vi "Measurement Logic.vi"() -> ()   [LabVIEW 2021, in "PWM Dimming.lvlib"]
uses:
  PWM Dimming.lvlib
  <vilib>/Plug-In SDKs/Measurements/Measure Call Context/Measure Call Context.lvclass
  Measurement Configuration.ctl
  Measurement Results.ctl
  Sub-VI/PWM measurement data.ctl
  <instrlib>/niDCPower/nidcpower.llb/niDCPower Source Mode.ctl
  <instrlib>/niDCPower/nidcpower.llb/niDCPower Output Function.ctl
  <instrlib>/niDCPower/nidcpower.llb/niDCPower Wait For Event - Event.ctl
  <instrlib>/niFgen/niFgen.llb/niFgen Output Mode.ctl
  <instrlib>/niFgen/niFgen.llb/niFgen Waveform Type.ctl
  <instrlib>/niDCPower/nidcpower.llb/niDCPower Aperture Time Units.ctl
  <instrlib>/niDCPower/nidcpower.llb/niDCPower Export Signal - Signal.ctl
  <instrlib>/niScope/Controls/niScope trigger slope.ctl
  <instrlib>/niFgen/niFgen.llb/niFgen Disable Start Trigger.vi
  <instrlib>/niDCPower/nidcpower.llb/niDCPower Configure Digital Edge Source Trigger With Channels.vi
  <instrlib>/niDCPower/nidcpower.llb/niDCPower Configure Digital Edge Measure Trigger With Channels.vi
  <instrlib>/niFgen/niFgen.llb/niFgen Configure Digital Edge Start Trigger.vi
  <instrlib>/niScope/Utility/niScope Get Channel Name From String.vi
  <instrlib>/niScope/Configure/Trigger/niScope Configure Trigger Digital.vi
  <instrlib>/niScope/Acquire/Fetch/niScope Fetch WDT.vi
panel:
  out "measurement results":T1
  in  "measurement configuration":T2={"DUT setup time"=1.0, "Nominal output voltage"=3.3, "Duty cycle single pulse/sweep pulse"=TRUE, "PWM frequency"=25.0, "Start duty cycle"=0.9, "Stop duty cycle"=99.1, "Number of sweep points"=10, "Duty cycle sweep type"="Linear", "Duty cycle single point"=50.0, "Number of pulse cycle"=10, "Source resource name"="", "Source sense"=1009, "Source voltage level"=12.0, "Source voltage level range"=15.0, "Source transient response"=1042, "Source voltage gain bandwidth"=2000.0, "Source voltage compensation frequency"=3530.0, "Source voltage pole-zero ratio"=2.0, "Load resource name"="", "Load sense"=1009, "Load pulse current level"=-0.02, "Load pulse bias current level"=0.0, "Load sample rate"=1800000.0, "Load voltage limit range"=15.0, "Load transient response"=1038, "Load current gain bandwidth"=50000.0, "Load current compensation frequency"=250000.0, "Load current pole-zero ratio"=5.0, "Source current limit range"=0.1, "AWG resource name"="0", "AWG channel name"="", "AWG amplitude"=4.0, "AWG dc offset"=2.0, "Scope resource name"="", "Scope input channel name"="0", "Scope sample rate"=1800000.0, "Scope probe attenuation"=10.0, "Scope vertical range"=15.0, "Scope vertical coupling"=enum."DC", "Load current level range"=15.0, "AWG load impedence"=100000.0, "Measurement timeout"=10.0, "AWG source trigger"="PFI0", "AWG measure trigger"=""} {"AWG load impedence" format="%.2f"; "Scope vertical range" format="%.2f"; "Scope probe attenuation" format="%.1f"; "Scope sample rate" step=1000000.0 format="%#.2g"; "AWG dc offset" format="%.2f"; "AWG amplitude" format="%.1f"; "Load transient response" items=["Slow"=1041, "Normal"=1038, "Fast"=1039, "Custom"=1042]; "Load pulse bias current level" format="%#_6p"; "Load pulse current level" format="%#_6p"; "Load sense" items=["Local"=1008, "Remote"=1009]; "Source transient response" items=["Slow"=1041, "Normal"=1038, "Fast"=1039, "Custom"=1042]; "Source sense" items=["Local"=1008, "Remote"=1009]}
  out "measure call context out":refnum<class "Measure Call Context.lvclass">
  in  "measure call context in":refnum<class "Measure Call Context.lvclass">
  out "error out":errorcluster
  in  "error in":errorcluster
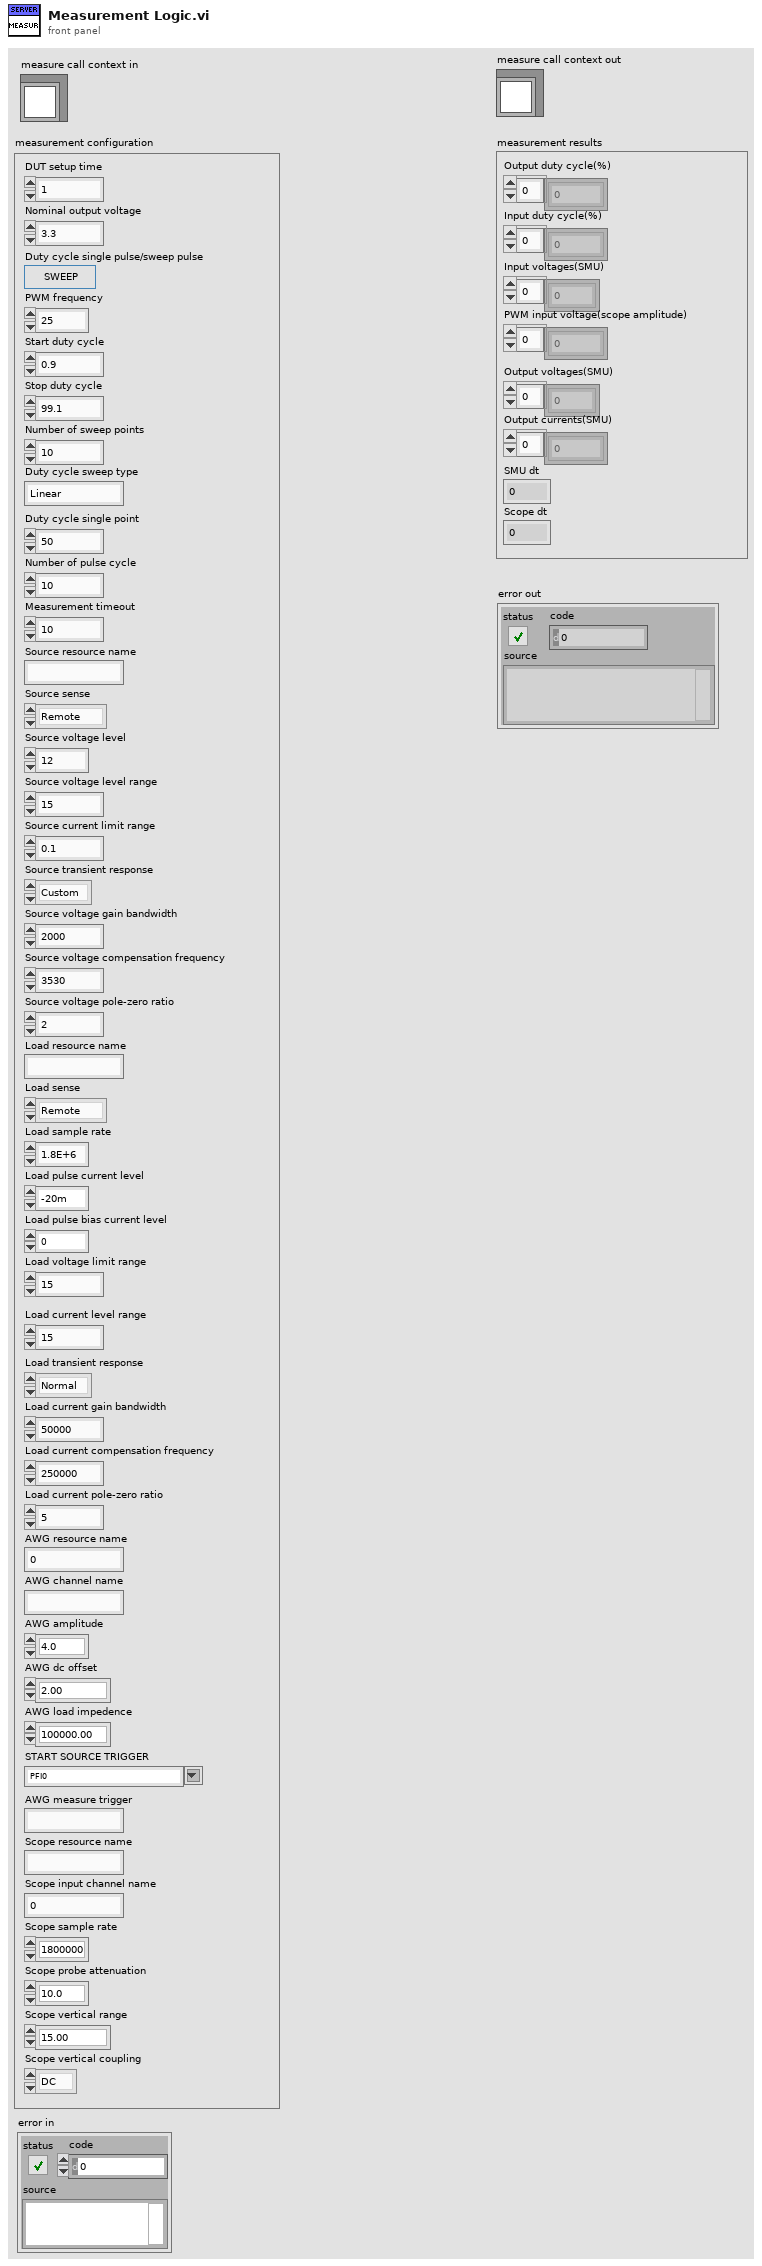
[diagram p1: front panel]
types:
  T1 = typedef "PWM Dimming.lvlib/Measurement Results.ctl" = cluster{"Output voltages(SMU)":dbl[], "Output currents(SMU)":dbl[], "Input voltages(SMU)":dbl[], "SMU dt":dbl, "Scope dt":dbl, "PWM input voltage(scope amplitude)":dbl[], "Output duty cycle(%)":dbl[], "Input duty cycle(%)":dbl[]}
  T2 = typedef "PWM Dimming.lvlib/Measurement Configuration.ctl" = cluster{"DUT setup time":dbl, "Nominal output voltage":dbl, "Duty cycle single pulse/sweep pulse":bool, "PWM frequency":dbl, "Start duty cycle":dbl, "Stop duty cycle":dbl, "Number of sweep points":i32, "Duty cycle sweep type":string, "Duty cycle single point":dbl, "Number of pulse cycle":i32, "Source resource name":string, "Source sense":i32, "Source voltage level":dbl, "Source voltage level range":dbl, "Source transient response":i32, "Source voltage gain bandwidth":dbl, "Source voltage compensation frequency":dbl, "Source voltage pole-zero ratio":dbl, "Load resource name":string, "Load sense":i32, "Load pulse current level":dbl, "Load pulse bias current level":dbl, "Load sample rate":dbl, "Load voltage limit range":dbl, "Load transient response":i32, "Load current gain bandwidth":dbl, "Load current compensation frequency":dbl, "Load current pole-zero ratio":dbl, "Source current limit range":dbl, "AWG resource name":string, "AWG channel name":string, "AWG amplitude":dbl, "AWG dc offset":dbl, "Scope resource name":string, "Scope input channel name":string, "Scope sample rate":dbl, "Scope probe attenuation":dbl, "Scope vertical range":dbl, "Scope vertical coupling":enum32{"AC", "DC"}, "Load current level range":dbl, "AWG load impedence":dbl, "Measurement timeout":dbl, "AWG source trigger":string, "AWG measure trigger":string}
  T3 = typedef "PWM measurement data.ctl" = cluster{"Source out":refnum<k15>, "Source channel name":string, "Load out":refnum<k15>, "Load channel name":string, "Source trigger terminal name":string, "Measure trigger terminal measure":string, "AWG Out":refnum<k15>, "scope channel name":string, "scope instrument handle out":refnum<k15>, "Measurement Results":T1, "No of samples to fetch smu single":i32, "No of samples to fetch scope single":i32, "Aperture Time":dbl, "Pulse On Time single":dbl, "Pulse Off Time single":dbl, "PWM voltage level":dbl, "Scope sample rate":dbl, "Frequency":dbl, "Load sample rate":dbl, "Current level absolute":dbl, "No of samples to fetch smu":i32, "No of samples to fetch scope":i32, "Pulse On Time":dbl, "Pulse Off Time":dbl, "Pulse current values":dbl[], "Frequency sweep values":dbl[], "Duty cycle index":i32}
  T4 = typedef "niDCPower Wait For Event - Event.ctl" = i32
  T5 = typedef "niDCPower Output Function.ctl" = i32
  T6 = typedef "niDCPower Source Mode.ctl" = i32
  T7 = typedef "niFgen Waveform Type.ctl" = i32
  T8 = typedef "niFgen Output Mode.ctl" = u32
  T9 = typedef "niDCPower Export Signal - Signal.ctl" = i32
  T10 = typedef "niDCPower Aperture Time Units.ctl" = i32
  T11 = typedef "niScope trigger slope.ctl" = i32
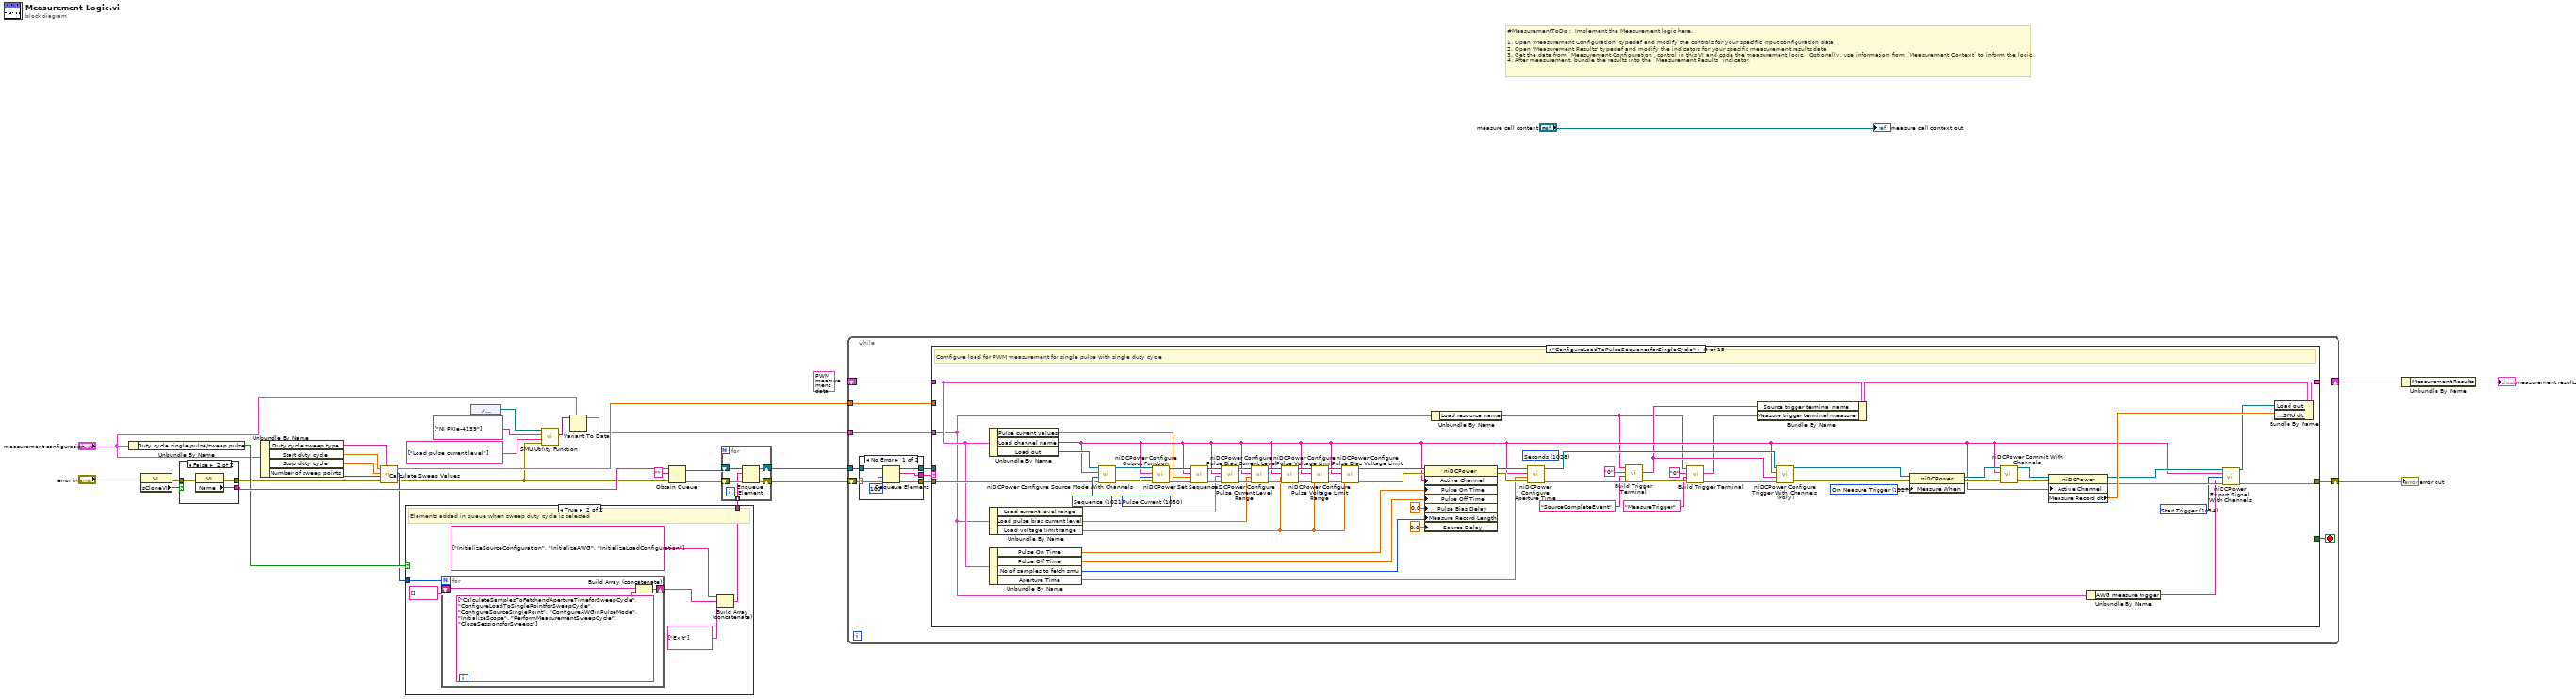
[diagram p0: block diagram]
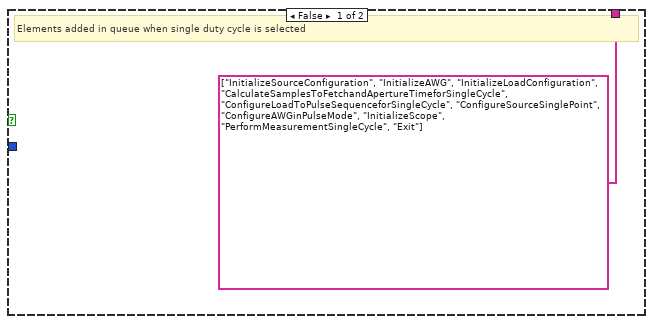
[diagram p2: hidden frame]
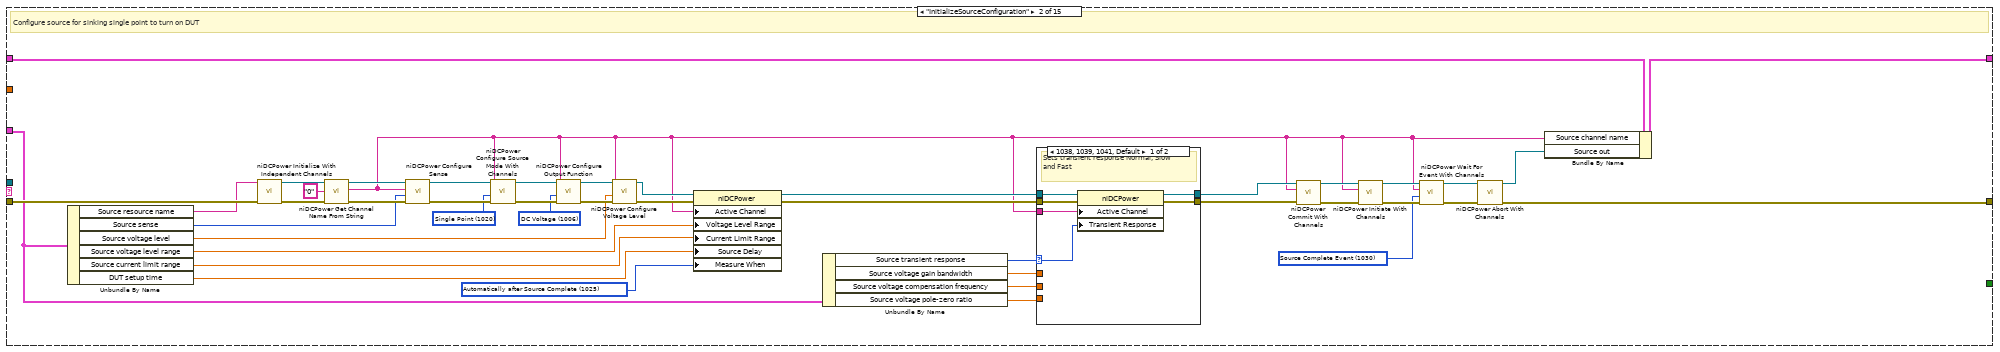
[diagram p4: hidden frame]
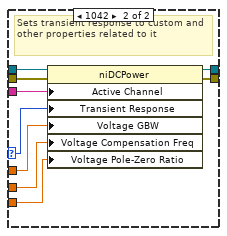
[diagram p5: hidden frame]
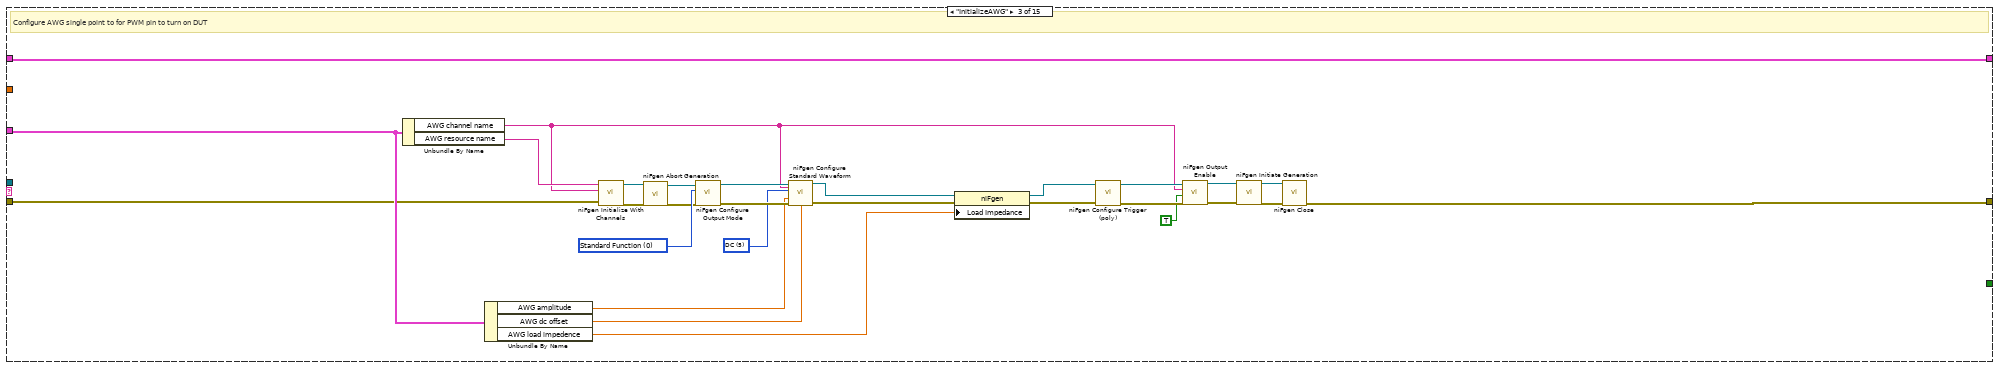
[diagram p6: hidden frame]
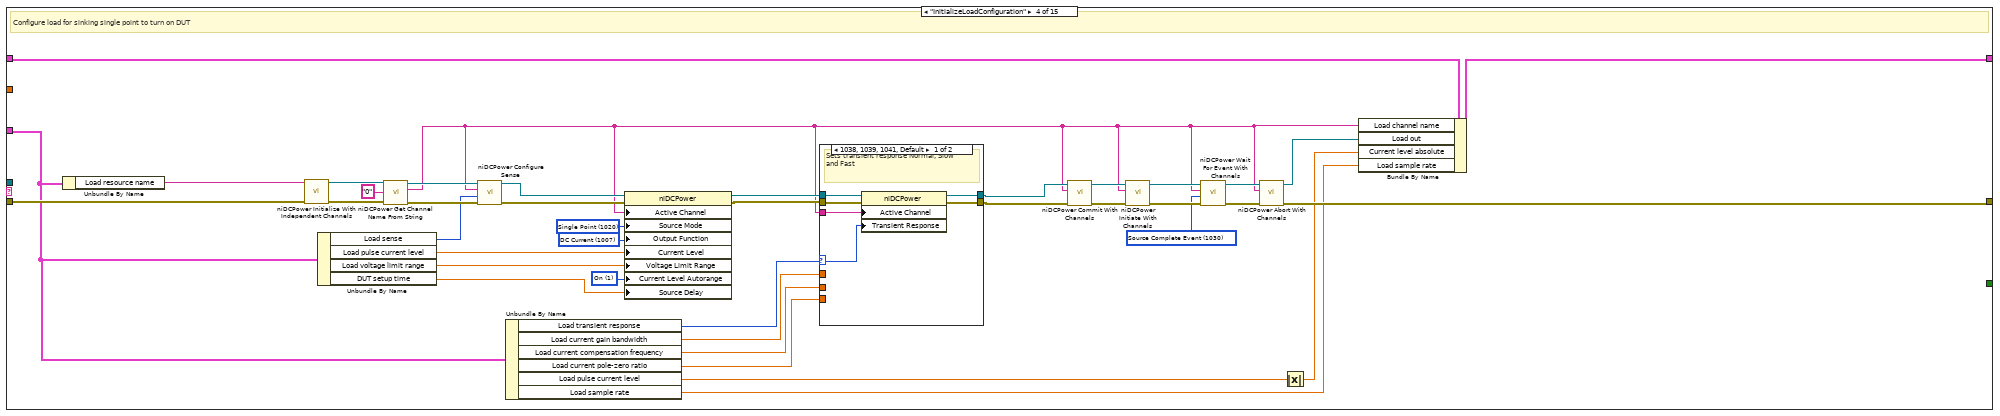
[diagram p7: hidden frame]
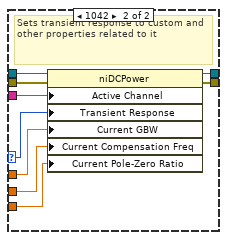
[diagram p8: hidden frame]
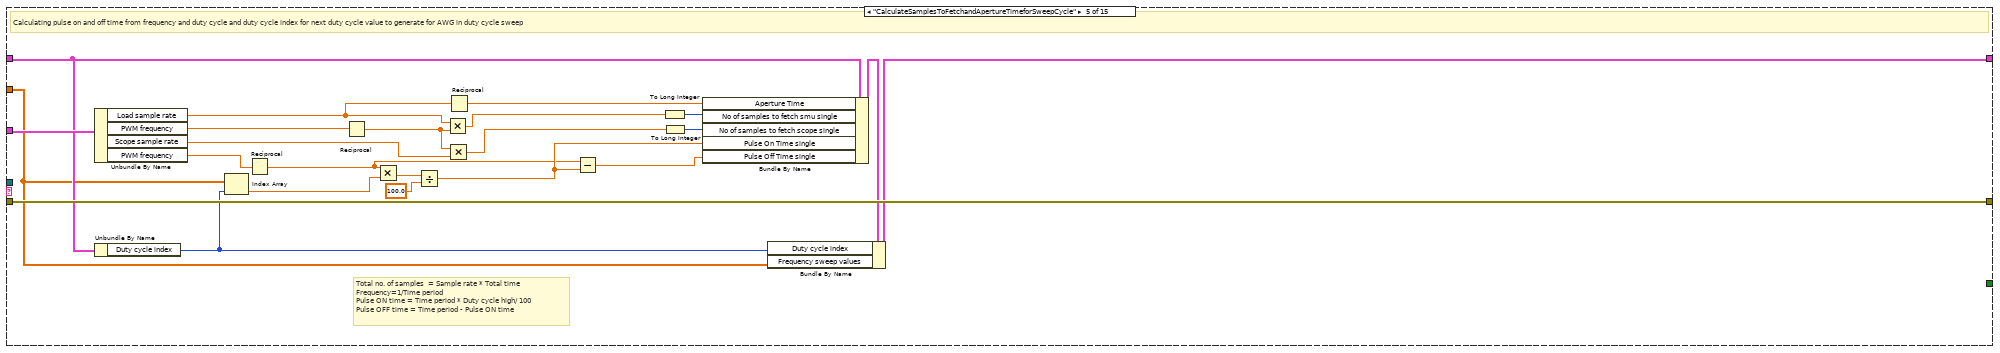
[diagram p9: hidden frame]
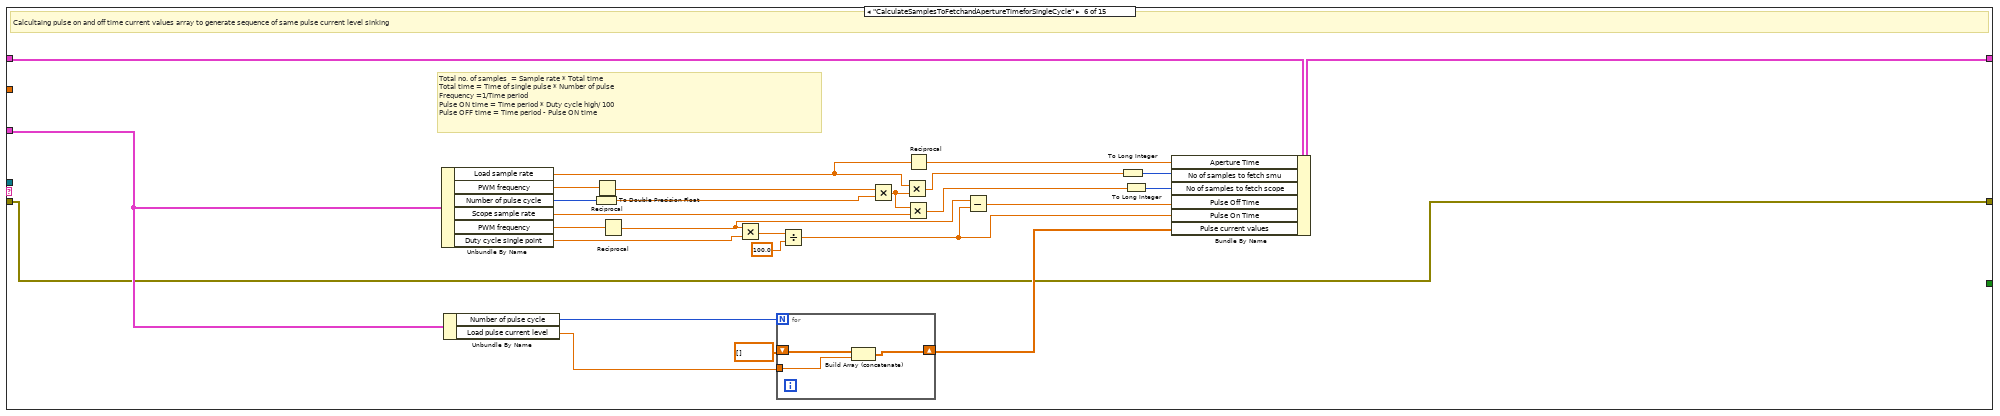
[diagram p10: hidden frame]
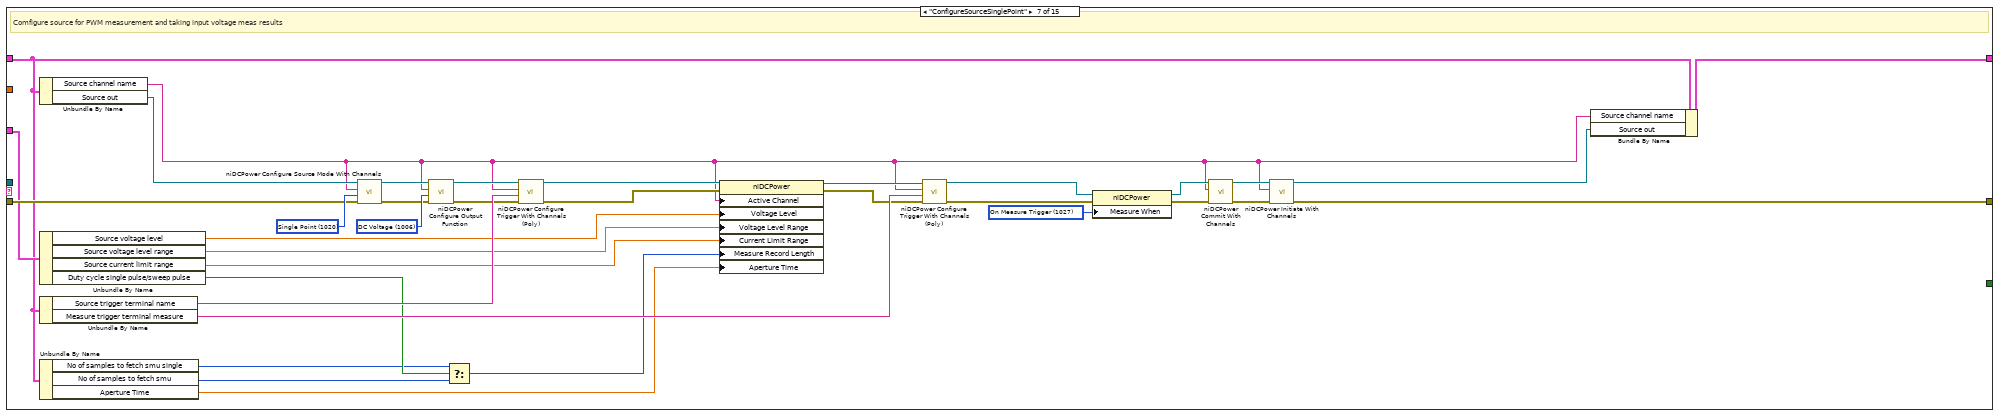
[diagram p11: hidden frame]
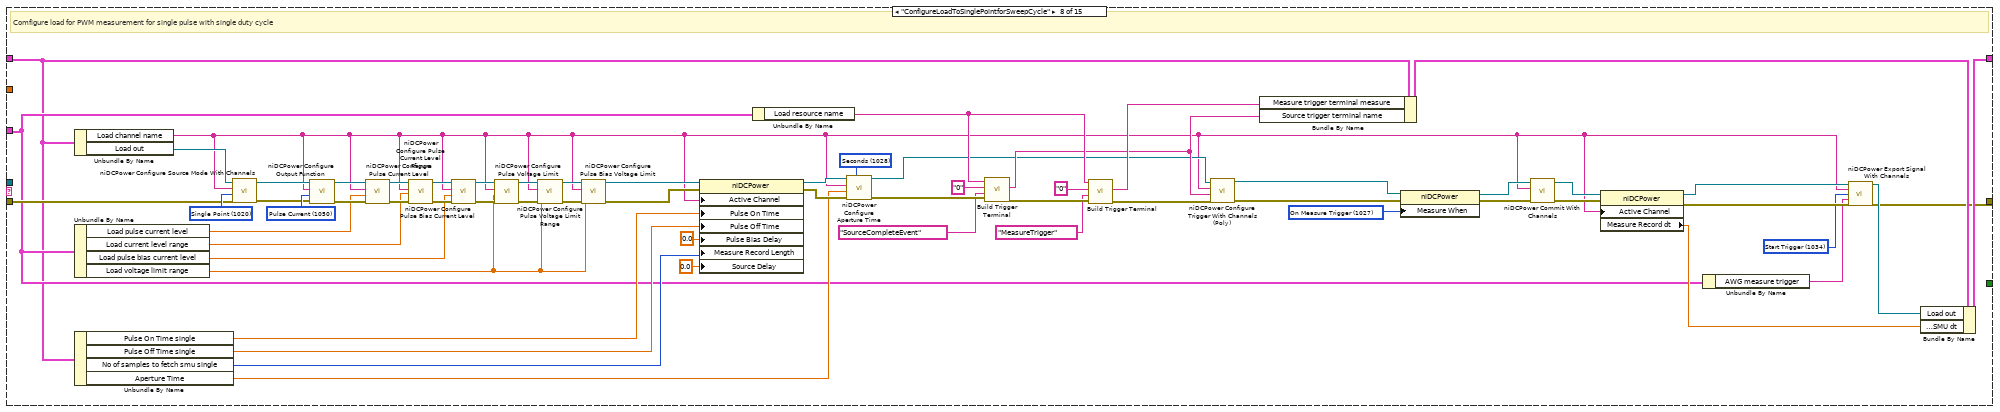
[diagram p12: hidden frame]
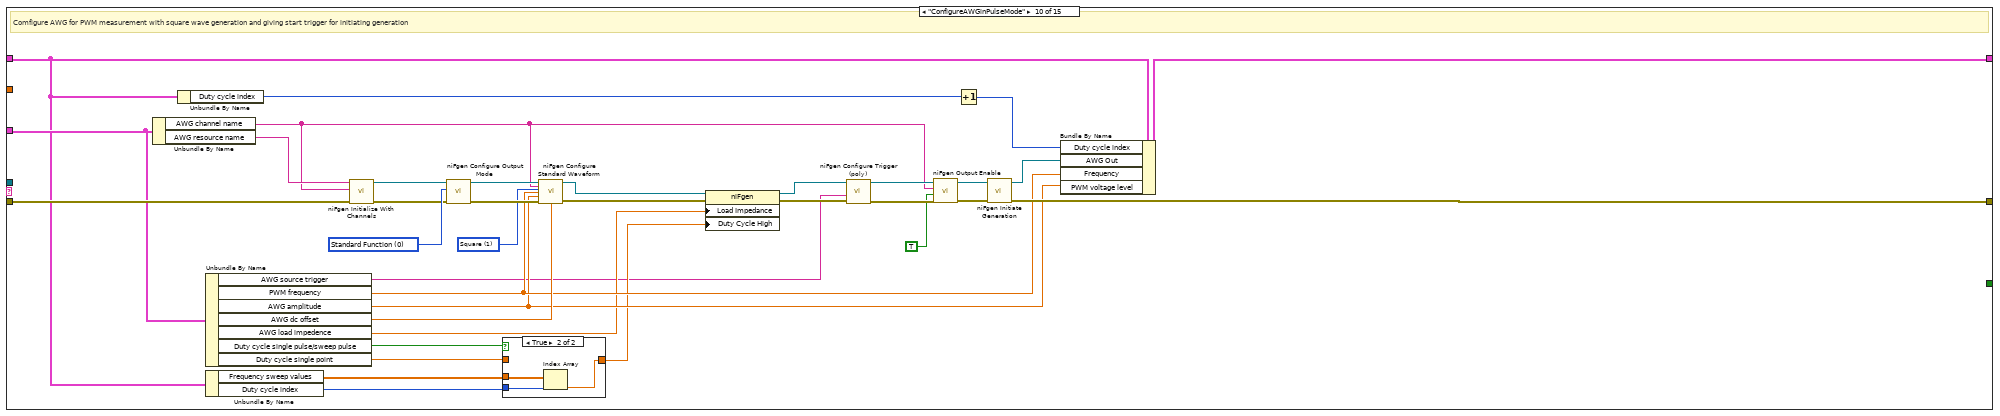
[diagram p13: hidden frame]
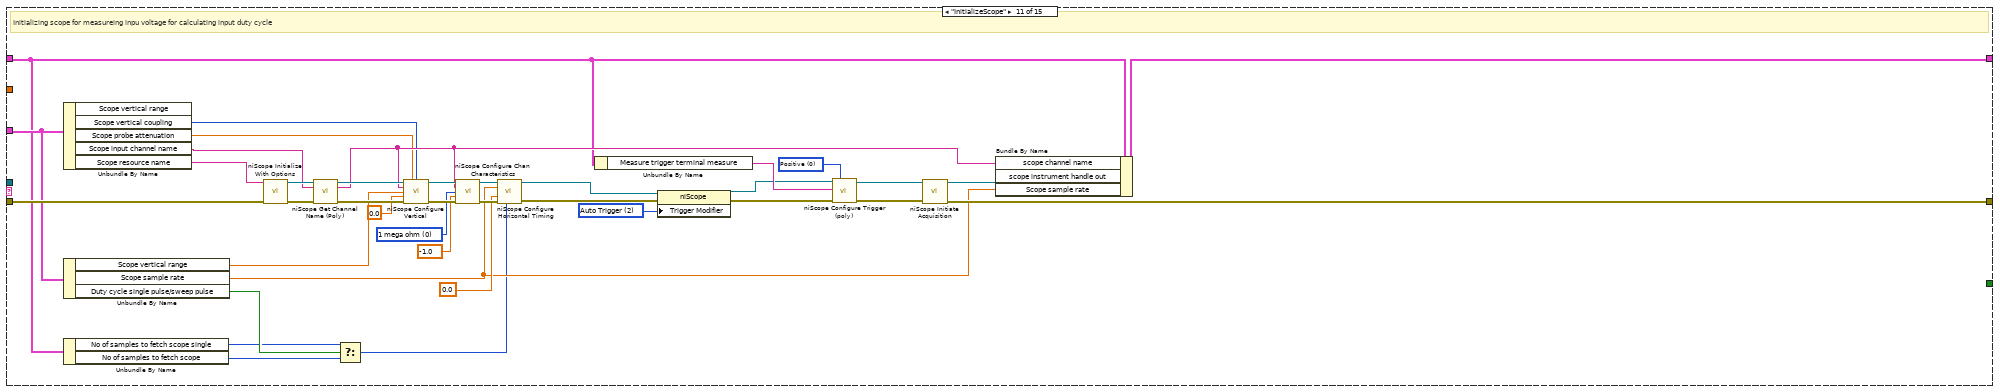
[diagram p15: hidden frame]
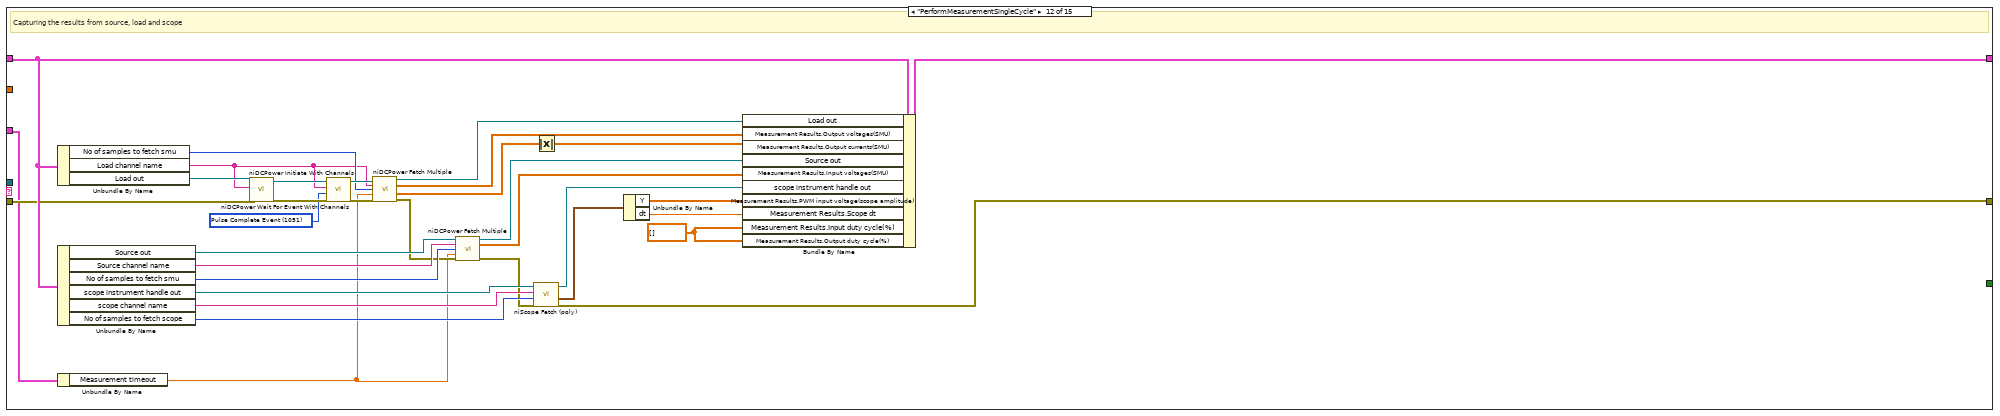
[diagram p16: hidden frame]
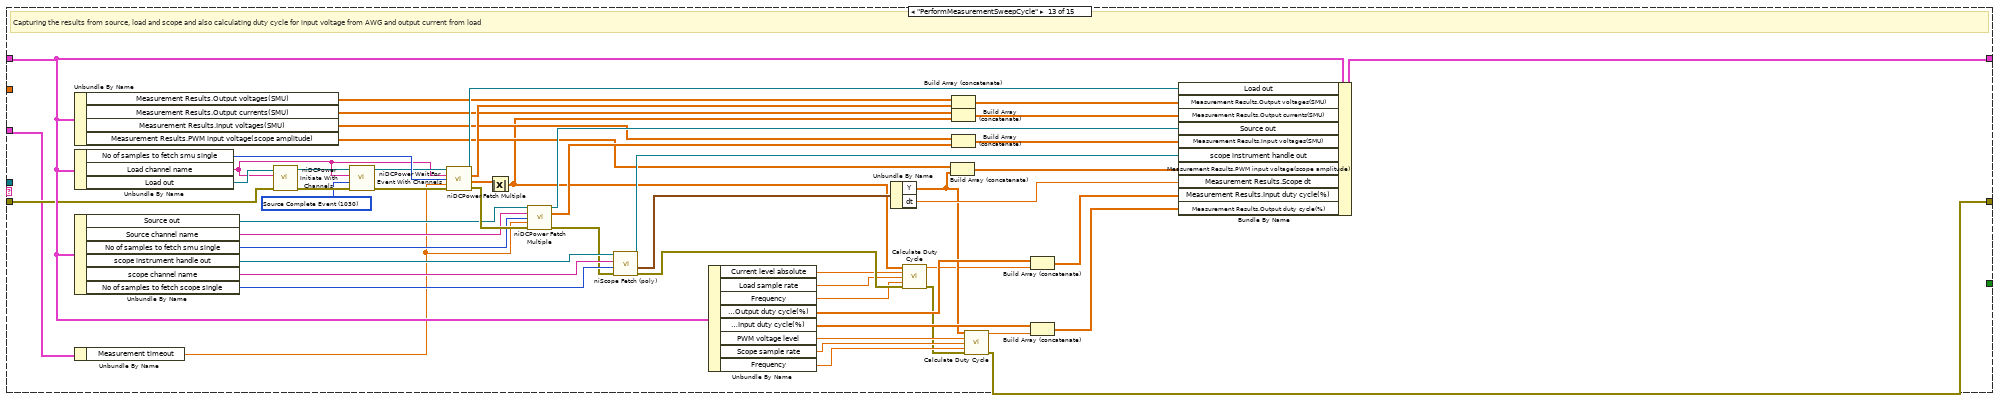
[diagram p17: hidden frame]
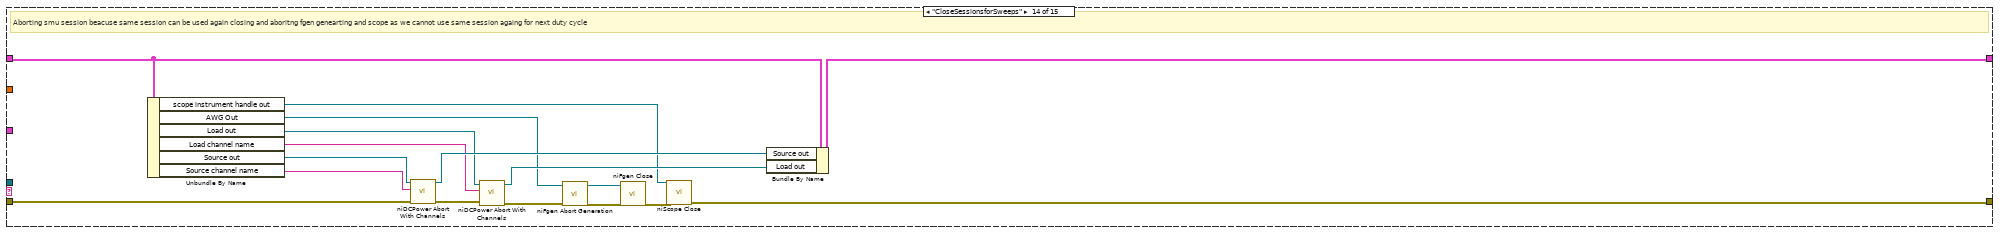
[diagram p18: hidden frame]
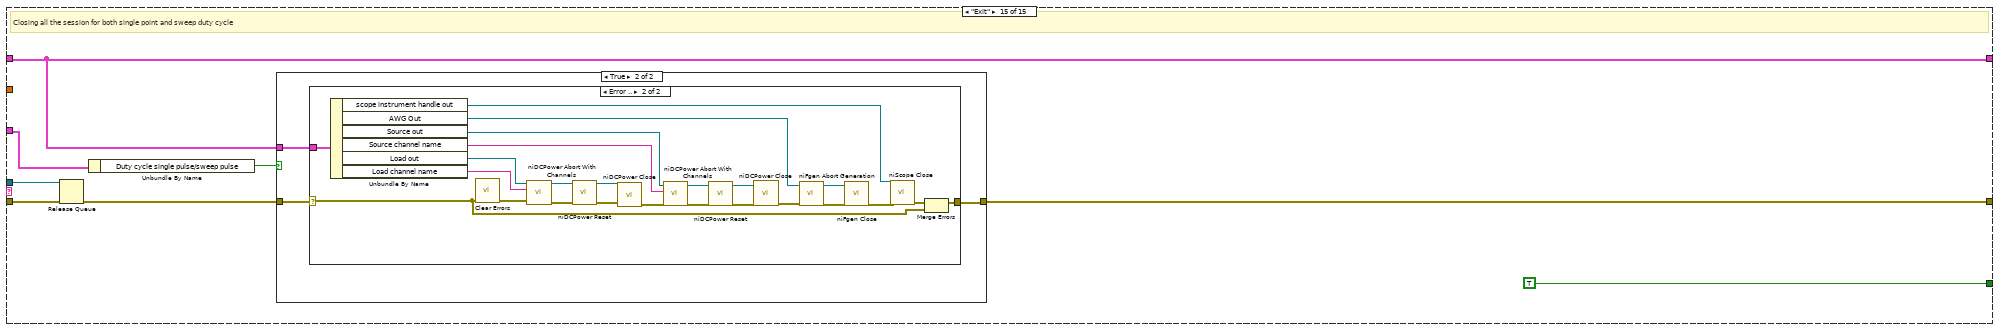
[diagram p19: hidden frame]
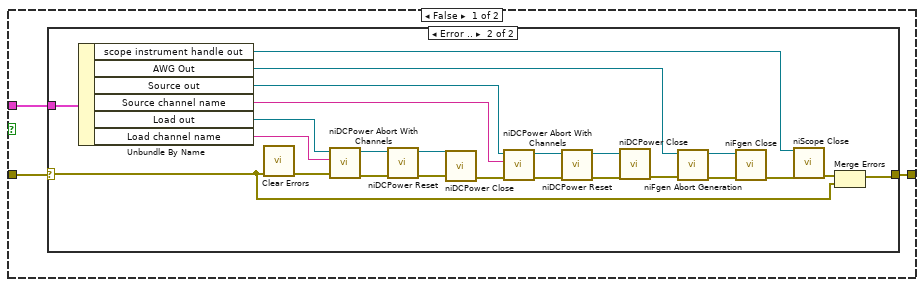
[diagram p20: hidden frame]
diagram:
  # "#MeasurementToDo :  Implement the Measurement logic here.\n\n1. Open 'Measurement Configuration' typedef and modify the controls for your specific input configuration data\n2. Open 'Measurement Results' typedef and modify the indicators for your specific measurement results data\n3. Get the data from `Measurement Configuration` control in this VI and code the measurement logic.  Optionally, use information from `Measurement Context` to inform the logic.\n4. After measurement, bundle the results into the `Measurement Results` indicator."
  n1 = Unbundle By Name("measurement configuration") -> ("Duty cycle single pulse/sweep pulse"=w16:bool)
  n2 = property class="VI"(error in="error in") -> (error out=w28:errorcluster, "IsCloneVI"=w29:bool)  [unwired: 1 in, 1 out]
  n3 = case shown="False" w29 {
    tunnel: [w33 w36] -> w15
    tunnel: [w32 w35] -> w26
    tunnel: w28 -> [w31 w34]
    frame True {
      n4 = property class="VI"(error in=w31) -> (error out=w33:errorcluster, "Clone Name"=w32:string)  [unwired: 1 in, 1 out]
    }
    frame False {
      n5 = property class="VI"(error in=w34) -> (error out=w36:errorcluster, "Name"=w35:string)  [unwired: 1 in, 1 out]
    }
  }
  n6 = Unbundle By Name("measurement configuration") -> ("Duty cycle sweep type"=w2:string, "Start duty cycle"=w3:dbl, "Stop duty cycle"=w4:dbl, "Number of sweep points"=w5:i32)
  n7 = call "Calculate Sweep Values.vi"("Sweep type"=w2, "error in"=w15, "Points"=w5, "Stop level"=w4, "Start level"=w3) -> ("error out"=w1:errorcluster, "Sweep points"=w14:i32, "Sweep values"=w13:dbl[])  [unwired: 4 in]
  n8 = case shown="True" w16 {
    tunnel: [string[] ["InitializeSourceConfiguration", "InitializeAWG", "InitializeLoadConfiguration", "CalculateSamplesToFetchandApertureTimeforSingleCycle", "ConfigureLoadToPulseSequenceforSingleCycle", "ConfigureSourceSinglePoint", "ConfigureAWGinPulseMode", "InitializeScope", "PerformMeasurementSingleCycle", "Exit"] ("Step sequence") w42] -> w18
    tunnel: w14 -> [_ w38]
    frame False {
      # "Elements added in queue when single duty cycle is selected"
    }
    frame True {
      # "Elements added in queue when sweep duty cycle is selected"
      n9 = for {
        N: w38 -> [_]
        shift-right: [w44] -> w41
        shift-left: string[] [] ("array") -> [w45]
        n10 = Build Array (concatenate)(w45, string[] ["CalculateSamplesToFetchandApertureTimeforSweepCycle", "ConfigureLoadToSinglePointforSweepCycle", "ConfigureSourceSinglePoint", "ConfigureAWGinPulseMode", "InitializeScope", "PerformMeasurementSweepCycle", "CloseSessionsforSweeps"] ("array")) -> (w44:string[])
      }
      n11 = Build Array (concatenate)(string[] ["InitializeSourceConfiguration", "InitializeAWG", "InitializeLoadConfiguration"] ("Step sequence"), w41, string[] ["Exit"] ("array")) -> (w42:string[])
    }
  }
  n12 = control-ref of="measurement configuration"() -> (w10:refnum<vi>)
  n13 = call "SMU Utility Function.vi"("error in"=w1, "Load Current Parameters"=string[] ["Load pulse current level"], "SMU Model"=string[] ["NI PXIe-4139"], "Measurement Configuration Ref"=w10) -> ("Measurement Configuration Out"=w12:variant)  [unwired: 6 in, 1 out]
  n14 = Variant To Data(type="measurement configuration", Variant=w12) -> (data=w7:T2)  [unwired: 1 in, 1 out]
  n15 = Obtain Queue(name (unnamed)=w26, element data type="", error in (no error)=w1) -> (queue out=w20:refnum<queue>, error out=w19:errorcluster)  [unwired: 2 in, 1 out]
  n16 = for {
    tunnel: w18 -> [w47] mode=indexing
    shift-right: [w50] -> w21
    shift-left: w20 -> [w49]
    shift-right: [w51] -> w22
    shift-left: w19 -> [w48]
    n17 = Enqueue Element(queue=w49, element=w47, error in (no error)=w48) -> (queue out=w50:refnum<queue>, error out=w51:errorcluster)  [unwired: 1 in, 1 out]
  }
  n18 = while {
    tunnel: w21 -> [w62]
    shift-right: [w55] -> w25
    shift-left: w22 -> [w61]
    tunnel: w7 -> [w57]
    shift-right: [w53] -> w17
    shift-left: T3 {"Source out"="", "Source channel name"="", "Load out"="", "Load channel name"="", "Source trigger terminal name"="", "Measure trigger terminal measure"="", "AWG Out"="", "scope channel name"="", "scope instrument handle out"="", "Measurement Results"={"Output voltages(SMU)"=[], "Output currents(SMU)"=[], "Input voltages(SMU)"=[], "SMU dt"=0.0, "Scope dt"=0.0, "PWM input voltage(scope amplitude)"=[], "Output duty cycle(%)"=[], "Input duty cycle(%)"=[]}, "No of samples to fetch smu single"=0, "No of samples to fetch scope single"=0, "Aperture Time"=0.0, "Pulse On Time single"=0.0, "Pulse Off Time single"=0.0, "PWM voltage level"=1.0, "Scope sample rate"=0.0, "Frequency"=0.0, "Load sample rate"=0.0, "Current level absolute"=1.0, "No of samples to fetch smu"=0, "No of samples to fetch scope"=0, "Pulse On Time"=0.0, "Pulse Off Time"=0.0, "Pulse current values"=[], "Frequency sweep values"=[], "Duty cycle index"=0} ("Cluster") -> [w54]
    tunnel: w13 -> [w52]
    stop <- w56 stop-if-true
    n19 = case shown="No Error" w61 {
      selector: w61 -> [w699 w703]
      tunnel: w62 -> [w701 w702]
      tunnel: [w700 "Exit" ("t")] -> w60
      tunnel: [w698 w703] -> w58
      tunnel: [w696 w702] -> w59
      frame No Error {
        n20 = Dequeue Element(queue=w701, timeout in ms (-1)=100, error in (no error)=w699) -> (queue out=w696:refnum<queue>, element=w700:string, error out=w698:errorcluster)  [unwired: 1 out]
      }
      frame Error {
      }
    }
    n21 = case shown="\"ConfigureLoadToPulseSequenceforSingleCycle\"" w60 {
      tunnel: w59 -> [_ _ _ _ _ _ _ _ _ _ _ _ _ _ w608]
      tunnel: w58 -> [w63 w92 w133 w179 w225 w235 w276 w312 w373 w450 w477 w507 w552 w585 w607]
      tunnel: w57 -> [_ w81 w134 w178 w216 w238 w274 w304 w362 w436 w470 w500 w545 _ w603]
      tunnel: [_ _ _ _ _ _ _ _ _ _ _ _ _ _ TRUE] -> w56
      tunnel: [w63 w67 w129 w157 w225 w235 w266 w296 w386 w439 w473 w524 w536 w591 w605] -> w55
      tunnel: w54 -> [w64 w91 w128 w176 w211 w237 w270 w302 w370 w426 w465 w529 w563 w596 w604]
      tunnel: [w64 w90 w128 w174 w212 w236 w269 w353 w359 w443 w476 w530 w564 w590 w604] -> w53
      tunnel: w52 -> [_ _ _ _ w210 _ _ _ _ _ _ _ _ _ _]
      frame Default {
      }
      frame "InitializeSourceConfiguration" {
        w66 = T4 1030 items=["Source Complete Event"=1030, "Measure Complete Event"=1031, "Sequence Iteration Complete Event"=1032, "Sequence Engine Done Event"=1033, "Pulse Complete Event"=1051, "Ready For Pulse Trigger Event"=1052] ("event")
        w73 = 1025 items=["Automatically after Source Complete"=1025, "On Demand"=1026, "On Measure Trigger"=1027] ("Measurement:Advanced:Measure When")
        w97 = T5 1006 items=["DC Voltage"=1006, "DC Current"=1007, "Pulse Voltage"=1049, "Pulse Current"=1050] ("output function")
        w98 = T6 1020 items=["Single Point"=1020, "Sequence"=1021] ("source mode")
        # "Configure source for sinking single point to turn on DUT"
        n22 = Unbundle By Name(w81) -> ("Source resource name"=w83:string, "Source sense"=w82:i32, "Source voltage level"=w85:dbl, "Source voltage level range"=w76:dbl, "Source current limit range"=w75:dbl, "DUT setup time"=w74:dbl)
        n23 = call <instrlib>:"niDCPower Initialize With Independent Channels.vi"("error in (no error)"=w92, "resource name"=w83) -> ("error out"=w87:errorcluster, "instrument handle out"=w89:refnum<k15>)  [unwired: 8 in]
        n24 = call <instrlib>:"niDCPower Get Channel Name From String.vi"("error in (no error)"=w87, "index"="0", "instrument handle"=w89) -> ("error out"=w86:errorcluster, "name"=w65:string, "instrument handle out"=w88:refnum<k15>)  [unwired: 6 in]
        n25 = call <instrlib>:"niDCPower Configure Sense.vi"("error in (no error)"=w86, "sense"=w82, "channel name"=w65, "instrument handle"=w88) -> ("error out"=w107:errorcluster, "instrument handle out"=w108:refnum<k15>)  [unwired: 6 in]
        n26 = call <instrlib>:"niDCPower Configure Source Mode With Channels.vi"("error in (no error)"=w107, "source mode"=w98, "channel name"=w65, "instrument handle"=w108) -> ("error out"=w99:errorcluster, "instrument handle out"=w100:refnum<k15>)  [unwired: 6 in]
        n27 = call <instrlib>:"niDCPower Configure Output Function.vi"("error in (no error)"=w99, "output function"=w97, "channel name"=w65, "instrument handle"=w100) -> ("error out"=w101:errorcluster, "instrument handle out"=w102:refnum<k15>)  [unwired: 6 in]
        n28 = call <instrlib>:"niDCPower Configure Voltage Level.vi"("error in (no error)"=w101, "voltage level"=w85, "channel name"=w65, "instrument handle"=w102) -> ("error out"=w104:errorcluster, "instrument handle out"=w103:refnum<k15>)  [unwired: 6 in]
        n29 = property class="niDCPower"(reference=w103, error in=w104, "Active Channel"=w65, "Voltage Level Range"=w76, "Current Limit Range"=w75, "Source Delay"=w74, "Measure When"=w73) -> (reference out=w96:refnum<k15>, error out=w94:errorcluster)
        n30 = Unbundle By Name(w81) -> ("Source transient response"=w80:i32, "Source voltage gain bandwidth"=w79:dbl, "Source voltage compensation frequency"=w78:dbl, "Source voltage pole-zero ratio"=w77:dbl)
        n31 = case shown="1038, 1039, 1041, Default" w80 {
          selector: w80 -> [w109 w116]
          tunnel: w96 -> [w114 w123]
          tunnel: [w113 w121] -> w95
          tunnel: w94 -> [w112 w122]
          tunnel: [w111 w120] -> w93
          tunnel: w65 -> [w110 w115]
          tunnel: w79 -> [_ w119]
          tunnel: w78 -> [_ w117]
          tunnel: w77 -> [_ w118]
          frame 1038, 1039, 1041, Default {
            # "Sets transient response Normal, Slow and Fast"
            n32 = property class="niDCPower"(reference=w114, error in=w112, "Active Channel"=w110, "Transient Response"=w109) -> (reference out=w113:refnum<k15>, error out=w111:errorcluster)
          }
          frame 1042 {
            # "Sets transient response to custom and other properties related to it"
            n33 = property class="niDCPower"(reference=w123, error in=w122, "Active Channel"=w115, "Transient Response"=w116, "Voltage GBW"=w119, "Voltage Compensation Freq"=w117, "Voltage Pole-Zero Ratio"=w118) -> (reference out=w121:refnum<k15>, error out=w120:errorcluster)
          }
        }
        n34 = call <instrlib>:"niDCPower Commit With Channels.vi"("error in (no error)"=w93, "channel name"=w65, "instrument handle"=w95) -> ("error out"=w106:errorcluster, "instrument handle out"=w105:refnum<k15>)  [unwired: 7 in]
        n35 = call <instrlib>:"niDCPower Initiate With Channels.vi"("error in (no error)"=w106, "channel name"=w65, "instrument handle"=w105) -> ("error out"=w69:errorcluster, "instrument handle out"=w70:refnum<k15>)  [unwired: 7 in]
        n36 = call <instrlib>:"niDCPower Wait For Event With Channels.vi"("error in (no error)"=w69, "event"=w66, "channel name"=w65, "instrument handle"=w70) -> ("error out"=w72:errorcluster, "instrument handle out"=w71:refnum<k15>)  [unwired: 6 in]
        n37 = call <instrlib>:"niDCPower Abort With Channels.vi"("error in (no error)"=w72, "instrument handle"=w71) -> ("error out"=w67:errorcluster, "instrument handle out"=w68:refnum<k15>)  [unwired: 8 in]
        n38 = Bundle By Name(cluster=w91, "Source channel name"=w65, "Source out"=w68) -> (w90:T3)
      }
      frame "InitializeAWG" {
        w148 = T7 5 items=["Sine", "Square", "Triangle", "Ramp Up", "Ramp Down", "DC", "Noise", "User"] ("Waveform")
        w149 = T8 0 items=["Standard Function", "Frequency List", "Arbitrary Waveform", "Arbitrary Sequence", "Script"] ("output mode")
        # "Configure AWG single point to for PWM pin to turn on DUT"
        n39 = Unbundle By Name(w134) -> ("AWG channel name"=w137:string, "AWG resource name"=w139:string)
        n40 = Unbundle By Name(w134) -> ("AWG amplitude"=w132:dbl, "AWG dc offset"=w138:dbl, "AWG load impedence"=w135:dbl)
        n41 = call <instrlib>:"niFgen Initialize With Channels.vi"("error in (no error)"=w133, "Channel Name"=w137, "Resource Name"=w139) -> ("error out"=w127:errorcluster, "Instrument Handle Out"=w125:refnum<k15>)  [unwired: 7 in]
        n42 = call <instrlib>:"niFgen Abort Generation.vi"("error in (no error)"=w127, "Instrument Handle"=w125) -> ("error out"=w126:errorcluster, "Instrument Handle Out"=w124:refnum<k15>)  [unwired: 8 in]
        n43 = call <instrlib>:"niFgen Configure Output Mode.vi"("error in (no error)"=w126, "Output Mode (default: 0=Standard Function)"=w149, "Instrument Handle"=w124) -> ("error out"=w151:errorcluster, "Instrument Handle Out"=w150:refnum<k15>)  [unwired: 6 in]
        n44 = call <instrlib>:"niFgen Configure Standard Waveform.vi"("Instrument Handle"=w150, "Channel Name"=w137, "Waveform"=w148, "Amplitude"=w132, "error in (no error)"=w151, "DC Offset"=w138) -> ("Instrument Handle Out"=w147:refnum<k15>, "error out"=w140:errorcluster)  [unwired: 8 in]
        n45 = property class="niFgen"(reference=w147, error in=w140, "Load Impedance"=w135) -> (reference out=w146:refnum<k15>, error out=w145:errorcluster)
        n46 = call-poly <instrlib>:"niFgen Configure Trigger (poly).vi"("error in (no error)"=w145, "Instrument Handle"=w146) -> ("error out"=w143:errorcluster, "Instrument Handle Out"=w144:refnum<k15>)  [unwired: 8 in]
        n47 = call <instrlib>:"niFgen Output Enable.vi"("error in (no error)"=w143, "Output Enable (default: True)"=TRUE ("output enable"), "Channel Name"=w137, "Instrument Handle"=w144) -> ("error out"=w142:errorcluster, "Instrument Handle Out"=w141:refnum<k15>)  [unwired: 6 in]
        n48 = call <instrlib>:"niFgen Initiate Generation.vi"("error in (no error)"=w142, "Instrument Handle"=w141) -> ("error out"=w131:errorcluster, "Instrument Handle Out"=w130:refnum<k15>)  [unwired: 8 in]
        n49 = call <instrlib>:"niFgen Close.vi"("error in (no error)"=w131, "Instrument Handle"=w130) -> ("error out"=w129:errorcluster)  [unwired: 9 in]
      }
      frame "InitializeLoadConfiguration" {
        w180 = 1 items=["Off", "On"] ("Source:DC Current:Current Level Autorange")
        w187 = T4 1030 items=["Source Complete Event"=1030, "Measure Complete Event"=1031, "Sequence Iteration Complete Event"=1032, "Sequence Engine Done Event"=1033, "Pulse Complete Event"=1051, "Ready For Pulse Trigger Event"=1052] ("event")
        w190 = 1007 items=["DC Voltage"=1006, "DC Current"=1007, "Pulse Voltage"=1049, "Pulse Current"=1050] ("Source:Output Function")
        w191 = 1020 items=["Single Point"=1020, "Sequence"=1021] ("Source:Source Mode")
        # "Configure load for sinking single point to turn on DUT"
        n50 = Unbundle By Name(w178) -> ("Load resource name"=w155:string)
        n51 = call <instrlib>:"niDCPower Initialize With Independent Channels.vi"("error in (no error)"=w179, "resource name"=w155) -> ("error out"=w170:errorcluster, "instrument handle out"=w168:refnum<k15>)  [unwired: 8 in]
        n52 = Unbundle By Name(w178) -> ("Load sense"=w169:i32, "Load pulse current level"=w167:dbl, "Load voltage limit range"=w173:dbl, "DUT setup time"=w177:dbl)
        n53 = call <instrlib>:"niDCPower Get Channel Name From String.vi"("error in (no error)"=w170, "index"="0", "instrument handle"=w168) -> ("error out"=w171:errorcluster, "name"=w158:string, "instrument handle out"=w172:refnum<k15>)  [unwired: 6 in]
        n54 = call <instrlib>:"niDCPower Configure Sense.vi"("error in (no error)"=w171, "sense"=w169, "channel name"=w158, "instrument handle"=w172) -> ("error out"=w183:errorcluster, "instrument handle out"=w184:refnum<k15>)  [unwired: 6 in]
        n55 = Unbundle By Name(w178) -> ("Load transient response"=w162:i32, "Load current gain bandwidth"=w161:dbl, "Load current compensation frequency"=w160:dbl, "Load current pole-zero ratio"=w159:dbl, "Load pulse current level"=w154:dbl, "Load sample rate"=w152:dbl)
        n56 = property class="niDCPower"(reference=w184, error in=w183, "Active Channel"=w158, "Source Mode"=w191, "Output Function"=w190, "Current Level"=w167, "Voltage Limit Range"=w173, "Current Level Autorange"=w180, "Source Delay"=w177) -> (reference out=w166:refnum<k15>, error out=w165:errorcluster)
        n57 = case shown="1038, 1039, 1041, Default" w162 {
          selector: w162 -> [w192 w199]
          tunnel: w166 -> [w197 w206]
          tunnel: [w196 w204] -> w164
          tunnel: w165 -> [w195 w205]
          tunnel: [w194 w203] -> w163
          tunnel: w158 -> [w193 w198]
          tunnel: w161 -> [_ w202]
          tunnel: w160 -> [_ w200]
          tunnel: w159 -> [_ w201]
          frame 1038, 1039, 1041, Default {
            # "Sets transient response Normal, Slow and Fast"
            n58 = property class="niDCPower"(reference=w197, error in=w195, "Active Channel"=w193, "Transient Response"=w192) -> (reference out=w196:refnum<k15>, error out=w194:errorcluster)
          }
          frame 1042 {
            # "Sets transient response to custom and other properties related to it"
            n59 = property class="niDCPower"(reference=w206, error in=w205, "Active Channel"=w198, "Transient Response"=w199, "Current GBW"=w202, "Current Compensation Freq"=w200, "Current Pole-Zero Ratio"=w201) -> (reference out=w204:refnum<k15>, error out=w203:errorcluster)
          }
        }
        n60 = call <instrlib>:"niDCPower Commit With Channels.vi"("error in (no error)"=w163, "channel name"=w158, "instrument handle"=w164) -> ("error out"=w181:errorcluster, "instrument handle out"=w182:refnum<k15>)  [unwired: 7 in]
        n61 = call <instrlib>:"niDCPower Initiate With Channels.vi"("error in (no error)"=w181, "channel name"=w158, "instrument handle"=w182) -> ("error out"=w189:errorcluster, "instrument handle out"=w188:refnum<k15>)  [unwired: 7 in]
        n62 = call <instrlib>:"niDCPower Wait For Event With Channels.vi"("error in (no error)"=w189, "event"=w187, "channel name"=w158, "instrument handle"=w188) -> ("error out"=w186:errorcluster, "instrument handle out"=w185:refnum<k15>)  [unwired: 6 in]
        n63 = call <instrlib>:"niDCPower Abort With Channels.vi"("error in (no error)"=w186, "channel name"=w158, "instrument handle"=w185) -> ("error out"=w157:errorcluster, "instrument handle out"=w175:refnum<k15>)  [unwired: 7 in]
        n64 = Absolute Value(x=w154) -> (abs(x)=w153:dbl)
        n65 = Bundle By Name(cluster=w176, "Load channel name"=w158, "Load out"=w175, "Current level absolute"=w153, "Load sample rate"=w152) -> (w174:T3)
      }
      frame "CalculateSamplesToFetchandApertureTimeforSweepCycle" {
        # "Total no. of samples  = Sample rate * Total time\nFrequency=1/Time period\nPulse ON time = Time period * Duty cycle high/ 100\nPulse OFF time = Time period - Pulse ON time"
        # "Calculating pulse on and off time from frequency and duty cycle and duty cycle index for next duty cycle value to generate for AWG in duty cycle sweep"
        n66 = Unbundle By Name(w216) -> ("Load sample rate"=w226:dbl, "PWM frequency"=w229:dbl, "Scope sample rate"=w227:dbl, "PWM frequency"=w219:dbl)
        n67 = Unbundle By Name(w211) -> ("Duty cycle index"=w209:i32)
        n68 = Index Array(array=w210, index=w209) -> (element=w208:dbl)
        n69 = Reciprocal(x=w219) -> (1/x=w207:dbl)
        n70 = Reciprocal(x=w229) -> (1/x=w228:dbl)
        n71 = Multiply(x=w207, y=w208) -> (x*y=w218:dbl)
        n72 = Divide(x=w218, y=100.0) -> (x/y=w214:dbl)
        n73 = Multiply(x=w226, y=w228) -> (x*y=w223:dbl)
        n74 = Multiply(x=w228, y=w227) -> (x*y=w221:dbl)
        n75 = Reciprocal(x=w226) -> (1/x=w224:dbl)
        n76 = Subtract(x=w207, y=w214) -> (x-y=w215:dbl)
        n77 = To Long Integer(number=w223) -> (32bit integer=w222:i32)
        n78 = To Long Integer(number=w221) -> (32bit integer=w220:i32)
        n79 = Bundle By Name(cluster=w211, "Aperture Time"=w224, "No of samples to fetch smu single"=w222, "No of samples to fetch scope single"=w220, "Pulse On Time single"=w214, "Pulse Off Time single"=w215) -> (w213:T3)
        n80 = Bundle By Name(cluster=w213, "Duty cycle index"=w209, "Frequency sweep values"=w210) -> (w212:T3)
      }
      frame "CalculateSamplesToFetchandApertureTimeforSingleCycle" {
        # "Total no. of samples  = Sample rate * Total time\nTotal time = Time of single pulse * Number of pulse\nFrequency =1/Time period\nPulse ON time = Time period * Duty cycle high/ 100\nPulse OFF time = Time period - Pulse ON time"
        # "Calcultaing pulse on and off time current values array to generate sequence of same pulse current level sinking"
        n81 = Unbundle By Name(w238) -> ("Load sample rate"=w252:dbl, "PWM frequency"=w256:dbl, "Number of pulse cycle"=w254:i32, "Scope sample rate"=w233:dbl, "PWM frequency"=w246:dbl, "Duty cycle single point"=w232:dbl)
        n82 = Unbundle By Name(w238) -> ("Number of pulse cycle"=w241:i32, "Load pulse current level"=w240:dbl)
        n83 = To Double Precision Float(number=w254) -> (double precision float=w234:dbl)
        n84 = Reciprocal(x=w256) -> (1/x=w255:dbl)
        n85 = Reciprocal(x=w246) -> (1/x=w243:dbl)
        n86 = Multiply(x=w243, y=w232) -> (x*y=w245:dbl)
        n87 = for {
          N: w241 -> [_]
          shift-right: [w258] -> w239
          shift-left: dbl[] [] ("array") -> [w259]
          tunnel: w240 -> [w257]
          n88 = Build Array (concatenate)(w259, w257) -> (w258:dbl[])
        }
        n89 = Divide(x=w245, y=100.0) -> (x/y=w230:dbl)
        n90 = Multiply(x=w255, y=w234) -> (x*y=w253:dbl)
        n91 = Multiply(x=w252, y=w253) -> (x*y=w250:dbl)
        n92 = Multiply(x=w253, y=w233) -> (x*y=w248:dbl)
        n93 = Reciprocal(x=w252) -> (1/x=w251:dbl)
        n94 = Subtract(x=w243, y=w230) -> (x-y=w231:dbl)
        n95 = To Long Integer(number=w250) -> (32bit integer=w249:i32)
        n96 = To Long Integer(number=w248) -> (32bit integer=w247:i32)
        n97 = Bundle By Name(cluster=w237, "Aperture Time"=w251, "No of samples to fetch smu"=w249, "No of samples to fetch scope"=w247, "Pulse Off Time"=w231, "Pulse On Time"=w230, "Pulse current values"=w239) -> (w236:T3)
      }
      frame "ConfigureSourceSinglePoint" {
        w281 = 1027 items=["Automatically after Source Complete"=1025, "On Demand"=1026, "On Measure Trigger"=1027] ("Measurement:Advanced:Measure When")
        w289 = T5 1006 items=["DC Voltage"=1006, "DC Current"=1007, "Pulse Voltage"=1049, "Pulse Current"=1050] ("output function")
        w288 = T6 1020 items=["Single Point"=1020, "Sequence"=1021] ("source mode")
        # "Comfigure source for PWM measurement and taking input voltage meas results"
        n98 = Unbundle By Name(w270) -> ("Source channel name"=w267:string, "Source out"=w275:refnum<k15>)
        n99 = Unbundle By Name(w274) -> ("Source voltage level"=w273:dbl, "Source voltage level range"=w261:dbl, "Source current limit range"=w260:dbl, "Duty cycle single pulse/sweep pulse"=w265:bool)
        n100 = Unbundle By Name(w270) -> ("Source trigger terminal name"=w294:string, "Measure trigger terminal measure"=w293:string)
        n101 = Unbundle By Name(w270) -> ("No of samples to fetch smu single"=w263:i32, "No of samples to fetch smu"=w264:i32, "Aperture Time"=w282:dbl)
        n102 = call <instrlib>:"niDCPower Configure Source Mode With Channels.vi"("error in (no error)"=w276, "source mode"=w288, "channel name"=w267, "instrument handle"=w275) -> ("error out"=w286:errorcluster, "instrument handle out"=w287:refnum<k15>)  [unwired: 6 in]
        n103 = call <instrlib>:"niDCPower Configure Output Function.vi"("error in (no error)"=w286, "output function"=w289, "channel name"=w267, "instrument handle"=w287) -> ("error out"=w291:errorcluster, "instrument handle out"=w290:refnum<k15>)  [unwired: 6 out]
        n104 = Select(t=w263, s=w265, f=w264) -> (s? t:f=w262:i32)
        n105 = call-poly <instrlib>:"niDCPower Configure Trigger With Channels (Poly).vi"("error in (no error)"=w291, "input terminal"=w294, "channel name"=w267, "instrument handle"=w290) -> ("error out"=w283:errorcluster, "instrument handle out"=w292:refnum<k15>)  [unwired: 6 in]
        n106 = property class="niDCPower"(reference=w292, error in=w283, "Active Channel"=w267, "Voltage Level"=w273, "Voltage Level Range"=w261, "Current Limit Range"=w260, "Measure Record Length"=w262, "Aperture Time"=w282) -> (reference out=w285:refnum<k15>, error out=w284:errorcluster)
        n107 = call-poly <instrlib>:"niDCPower Configure Trigger With Channels (Poly).vi"("error in (no error)"=w284, "input terminal"=w293, "channel name"=w267, "instrument handle"=w285) -> ("error out"=w280:errorcluster, "instrument handle out"=w278:refnum<k15>)  [unwired: 6 in]
        n108 = property class="niDCPower"(reference=w278, error in=w280, "Measure When"=w281) -> (reference out=w277:refnum<k15>, error out=w279:errorcluster)
        n109 = call <instrlib>:"niDCPower Commit With Channels.vi"("error in (no error)"=w279, "channel name"=w267, "instrument handle"=w277) -> ("error out"=w272:errorcluster, "instrument handle out"=w271:refnum<k15>)  [unwired: 7 in]
        n110 = call <instrlib>:"niDCPower Initiate With Channels.vi"("error in (no error)"=w272, "channel name"=w267, "instrument handle"=w271) -> ("error out"=w266:errorcluster, "instrument handle out"=w268:refnum<k15>)  [unwired: 7 in]
        n111 = Bundle By Name(cluster=w270, "Source channel name"=w267, "Source out"=w268) -> (w269:T3)
      }
      frame "ConfigureLoadToSinglePointforSweepCycle" {
        w322 = T9 1034 items=["Source Complete Event"=1030, "Measure Complete Event"=1031, "Sequence Iteration Complete Event"=1032, "Sequence Engine Done Event"=1033, "Pulse Complete Event"=1051, "Ready For Pulse Trigger Event"=1052, "Start Trigger"=1034, "Source Trigger"=1035, "Measure Trigger"=1036, "Sequence Advance Trigger"=1037, "Pulse Trigger"=1053] ("signal")
        w332 = T5 1050 items=["DC Voltage"=1006, "DC Current"=1007, "Pulse Voltage"=1049, "Pulse Current"=1050] ("output function")
        w342 = T10 1028 items=["Seconds"=1028, "Powerline Cycles"=1029] ("aperture time units")
        w351 = 1027 items=["Automatically after Source Complete"=1025, "On Demand"=1026, "On Measure Trigger"=1027] ("Measurement:Advanced:Measure When")
        w355 = T6 1020 items=["Single Point"=1020, "Sequence"=1021] ("source mode")
        # "Comfigure load for PWM measurement for single pulse with single duty cycle"
        n112 = Unbundle By Name(w302) -> ("Load channel name"=w295:string, "Load out"=w354:refnum<k15>)
        n113 = Unbundle By Name(w304) -> ("Load pulse current level"=w313:dbl, "Load current level range"=w321:dbl, "Load pulse bias current level"=w320:dbl, "Load voltage limit range"=w319:dbl)
        n114 = Unbundle By Name(w302) -> ("Pulse On Time single"=w318:dbl, "Pulse Off Time single"=w317:dbl, "No of samples to fetch smu single"=w316:i32, "Aperture Time"=w315:dbl)
        n115 = call <instrlib>:"niDCPower Configure Source Mode With Channels.vi"("error in (no error)"=w312, "source mode"=w355, "channel name"=w295, "instrument handle"=w354) -> ("error out"=w328:errorcluster, "instrument handle out"=w327:refnum<k15>)  [unwired: 6 in]
        n116 = call <instrlib>:"niDCPower Configure Output Function.vi"("error in (no error)"=w328, "output function"=w332, "channel name"=w295, "instrument handle"=w327) -> ("error out"=w331:errorcluster, "instrument handle out"=w330:refnum<k15>)  [unwired: 6 out]
        n117 = call <instrlib>:"niDCPower Configure Pulse Current Level.vi"("error in (no error)"=w331, "pulse current level"=w313, "channel name"=w295, "instrument handle"=w330) -> ("error out"=w341:errorcluster, "instrument handle out"=w329:refnum<k15>)  [unwired: 6 in]
        n118 = call <instrlib>:"niDCPower Configure Pulse Current Level Range.vi"("error in (no error)"=w341, "pulse current level range"=w321, "channel name"=w295, "instrument handle"=w329) -> ("error out"=w340:errorcluster, "instrument handle out"=w339:refnum<k15>)  [unwired: 6 in]
        n119 = call <instrlib>:"niDCPower Configure Pulse Bias Current Level.vi"("error in (no error)"=w340, "pulse bias current level"=w320, "channel name"=w295, "instrument handle"=w339) -> ("error out"=w338:errorcluster, "instrument handle out"=w337:refnum<k15>)  [unwired: 6 in]
        n120 = call <instrlib>:"niDCPower Configure Pulse Voltage Limit.vi"("error in (no error)"=w338, "pulse voltage limit"=w319, "channel name"=w295, "instrument handle"=w337) -> ("error out"=w336:errorcluster, "instrument handle out"=w335:refnum<k15>)  [unwired: 6 in]
        n121 = call <instrlib>:"niDCPower Configure Pulse Voltage Limit Range.vi"("error in (no error)"=w336, "pulse voltage limit range"=w319, "channel name"=w295, "instrument handle"=w335) -> ("error out"=w334:errorcluster, "instrument handle out"=w333:refnum<k15>)  [unwired: 6 in]
        n122 = call <instrlib>:"niDCPower Configure Pulse Bias Voltage Limit.vi"("error in (no error)"=w334, "pulse bias voltage limit"=w319, "channel name"=w295, "instrument handle"=w333) -> ("error out"=w345:errorcluster, "instrument handle out"=w346:refnum<k15>)  [unwired: 6 in]
        n123 = property class="niDCPower"(reference=w346, error in=w345, "Active Channel"=w295, "Pulse On Time"=w318, "Pulse Off Time"=w317, "Pulse Bias Delay"=0.0 ("Source:Advanced:Pulse Bias Delay"), "Measure Record Length"=w316, "Source Delay"=0.0 ("Source:Advanced:Source Delay")) -> (reference out=w343:refnum<k15>, error out=w344:errorcluster)
        n124 = Unbundle By Name(w304) -> ("Load resource name"=w303:string)
        n125 = call <instrlib>:"niDCPower Configure Aperture Time.vi"("aperture time units"=w342, "error in (no error)"=w344, "aperture time"=w315, "channel name"=w295, "instrument handle"=w343) -> ("error out"=w309:errorcluster, "instrument handle out"=w298:refnum<k15>)  [unwired: 5 in]
        n126 = call "Build Trigger Terminal.vi"("error in (no error)"=w309, "Trigger/Event Name"="SourceCompleteEvent", "Channel Name"="0", "Resource Name"=w303) -> ("error out"=w311:errorcluster, "Terminal Name"=w299:string)  [unwired: 6 in]
        n127 = call "Build Trigger Terminal.vi"("error in (no error)"=w311, "Trigger/Event Name"="MeasureTrigger", "Channel Name"="0", "Resource Name"=w303) -> ("error out"=w308:errorcluster, "Terminal Name"=w300:string)  [unwired: 6 in]
        n128 = call-poly <instrlib>:"niDCPower Configure Trigger With Channels (Poly).vi"("error in (no error)"=w308, "input terminal"=w299, "channel name"=w295, "instrument handle"=w298) -> ("error out"=w348:errorcluster, "instrument handle out"=w350:refnum<k15>)  [unwired: 6 in]
        n129 = Bundle By Name(cluster=w302, "Measure trigger terminal measure"=w300, "Source trigger terminal name"=w299) -> (w301:T3)
        n130 = property class="niDCPower"(reference=w350, error in=w348, "Measure When"=w351) -> (reference out=w349:refnum<k15>, error out=w347:errorcluster)
        n131 = call <instrlib>:"niDCPower Commit With Channels.vi"("error in (no error)"=w347, "channel name"=w295, "instrument handle"=w349) -> ("error out"=w357:errorcluster, "instrument handle out"=w356:refnum<k15>)  [unwired: 7 in]
        n132 = property class="niDCPower"(reference=w356, error in=w357, "Active Channel"=w295) -> (reference out=w323:refnum<k15>, error out=w324:errorcluster, "Measure Record dt"=w352:dbl)
        n133 = Unbundle By Name(w304) -> ("AWG measure trigger"=w314:string)
        n134 = call <instrlib>:"niDCPower Export Signal With Channels.vi"("instrument handle"=w323, "channel name"=w295, "signal"=w322, "output terminal"=w314, "error in (no error)"=w324) -> ("instrument handle out"=w297:refnum<k15>, "error out"=w296:errorcluster)  [unwired: 9 in]
        n135 = Bundle By Name(cluster=w301, "Load out"=w297, "Measurement Results.SMU dt"=w352) -> (w353:T3)
      }
      frame "ConfigureLoadToPulseSequenceforSingleCycle" {
        w382 = T9 1034 items=["Source Complete Event"=1030, "Measure Complete Event"=1031, "Sequence Iteration Complete Event"=1032, "Sequence Engine Done Event"=1033, "Pulse Complete Event"=1051, "Ready For Pulse Trigger Event"=1052, "Start Trigger"=1034, "Source Trigger"=1035, "Measure Trigger"=1036, "Sequence Advance Trigger"=1037, "Pulse Trigger"=1053] ("signal")
        w396 = T5 1050 items=["DC Voltage"=1006, "DC Current"=1007, "Pulse Voltage"=1049, "Pulse Current"=1050] ("output function")
        w406 = T10 1028 items=["Seconds"=1028, "Powerline Cycles"=1029] ("aperture time units")
        w415 = 1027 items=["Automatically after Source Complete"=1025, "On Demand"=1026, "On Measure Trigger"=1027] ("Measurement:Advanced:Measure When")
        w418 = T6 1021 items=["Single Point"=1020, "Sequence"=1021] ("source mode")
        # "Comfigure load for PWM measurement for single pulse with single duty cycle"
        n136 = Unbundle By Name(w370) -> ("Pulse current values"=w381:dbl[], "Load channel name"=w383:string, "Load out"=w417:refnum<k15>)
        n137 = Unbundle By Name(w362) -> ("Load current level range"=w380:dbl, "Load pulse bias current level"=w379:dbl, "Load voltage limit range"=w378:dbl)
        n138 = Unbundle By Name(w370) -> ("Pulse On Time"=w377:dbl, "Pulse Off Time"=w376:dbl, "No of samples to fetch smu"=w375:i32, "Aperture Time"=w374:dbl)
        n139 = call <instrlib>:"niDCPower Configure Source Mode With Channels.vi"("error in (no error)"=w373, "source mode"=w418, "channel name"=w383, "instrument handle"=w417) -> ("error out"=w392:errorcluster, "instrument handle out"=w391:refnum<k15>)  [unwired: 6 in]
        n140 = call <instrlib>:"niDCPower Configure Output Function.vi"("error in (no error)"=w392, "output function"=w396, "channel name"=w383, "instrument handle"=w391) -> ("error out"=w395:errorcluster, "instrument handle out"=w394:refnum<k15>)  [unwired: 6 out]
        n141 = call <instrlib>:"niDCPower Set Sequence.vi"("error in (no error)"=w395, "values"=w381, "channel name"=w383, "instrument handle"=w394) -> ("error out"=w405:errorcluster, "instrument handle out"=w393:refnum<k15>)  [unwired: 6 in]
        n142 = call <instrlib>:"niDCPower Configure Pulse Current Level Range.vi"("error in (no error)"=w405, "pulse current level range"=w380, "channel name"=w383, "instrument handle"=w393) -> ("error out"=w404:errorcluster, "instrument handle out"=w403:refnum<k15>)  [unwired: 6 in]
        n143 = call <instrlib>:"niDCPower Configure Pulse Bias Current Level.vi"("error in (no error)"=w404, "pulse bias current level"=w379, "channel name"=w383, "instrument handle"=w403) -> ("error out"=w402:errorcluster, "instrument handle out"=w401:refnum<k15>)  [unwired: 6 in]
        n144 = call <instrlib>:"niDCPower Configure Pulse Voltage Limit.vi"("error in (no error)"=w402, "pulse voltage limit"=w378, "channel name"=w383, "instrument handle"=w401) -> ("error out"=w400:errorcluster, "instrument handle out"=w399:refnum<k15>)  [unwired: 6 in]
        n145 = call <instrlib>:"niDCPower Configure Pulse Voltage Limit Range.vi"("error in (no error)"=w400, "pulse voltage limit range"=w378, "channel name"=w383, "instrument handle"=w399) -> ("error out"=w398:errorcluster, "instrument handle out"=w397:refnum<k15>)  [unwired: 6 in]
        n146 = call <instrlib>:"niDCPower Configure Pulse Bias Voltage Limit.vi"("error in (no error)"=w398, "pulse bias voltage limit"=w378, "channel name"=w383, "instrument handle"=w397) -> ("error out"=w409:errorcluster, "instrument handle out"=w410:refnum<k15>)  [unwired: 6 in]
        n147 = property class="niDCPower"(reference=w410, error in=w409, "Active Channel"=w383, "Pulse On Time"=w377, "Pulse Off Time"=w376, "Pulse Bias Delay"=0.0 ("Source:Advanced:Pulse Bias Delay"), "Measure Record Length"=w375, "Source Delay"=0.0 ("Source:Advanced:Source Delay")) -> (reference out=w407:refnum<k15>, error out=w408:errorcluster)
        n148 = Unbundle By Name(w362) -> ("Load resource name"=w361:string)
        n149 = call <instrlib>:"niDCPower Configure Aperture Time.vi"("aperture time units"=w406, "error in (no error)"=w408, "aperture time"=w374, "channel name"=w383, "instrument handle"=w407) -> ("error out"=w366:errorcluster, "instrument handle out"=w390:refnum<k15>)  [unwired: 5 in]
        n150 = call "Build Trigger Terminal.vi"("error in (no error)"=w366, "Trigger/Event Name"="SourceCompleteEvent", "Channel Name"="0", "Resource Name"=w361) -> ("error out"=w372:errorcluster, "Terminal Name"=w368:string)  [unwired: 6 in]
        n151 = call "Build Trigger Terminal.vi"("error in (no error)"=w372, "Trigger/Event Name"="MeasureTrigger", "Channel Name"="0", "Resource Name"=w361) -> ("error out"=w365:errorcluster, "Terminal Name"=w367:string)  [unwired: 6 in]
        n152 = Bundle By Name(cluster=w370, "Source trigger terminal name"=w368, "Measure trigger terminal measure"=w367) -> (w369:T3)
        n153 = call-poly <instrlib>:"niDCPower Configure Trigger With Channels (Poly).vi"("error in (no error)"=w365, "input terminal"=w368, "channel name"=w383, "instrument handle"=w390) -> ("error out"=w412:errorcluster, "instrument handle out"=w414:refnum<k15>)  [unwired: 6 in]
        n154 = property class="niDCPower"(reference=w414, error in=w412, "Measure When"=w415) -> (reference out=w413:refnum<k15>, error out=w411:errorcluster)
        n155 = call <instrlib>:"niDCPower Commit With Channels.vi"("error in (no error)"=w411, "channel name"=w383, "instrument handle"=w413) -> ("error out"=w420:errorcluster, "instrument handle out"=w419:refnum<k15>)  [unwired: 7 in]
        n156 = property class="niDCPower"(reference=w419, error in=w420, "Active Channel"=w383) -> (reference out=w385:refnum<k15>, error out=w387:errorcluster, "Measure Record dt"=w416:dbl)
        n157 = Unbundle By Name(w362) -> ("AWG measure trigger"=w358:string)
        n158 = call <instrlib>:"niDCPower Export Signal With Channels.vi"("instrument handle"=w385, "channel name"=w383, "signal"=w382, "output terminal"=w358, "error in (no error)"=w387) -> ("instrument handle out"=w384:refnum<k15>, "error out"=w386:errorcluster)  [unwired: 9 in]
        n159 = Bundle By Name(cluster=w369, "Load out"=w384, "Measurement Results.SMU dt"=w416) -> (w359:T3)
      }
      frame "ConfigureAWGinPulseMode" {
        w449 = T7 1 items=["Sine", "Square", "Triangle", "Ramp Up", "Ramp Down", "DC", "Noise", "User"] ("Waveform")
        w453 = T8 0 items=["Standard Function", "Frequency List", "Arbitrary Waveform", "Arbitrary Sequence", "Script"] ("output mode")
        # "Comfigure AWG for PWM measurement with square wave generation and giving start trigger for initiating generation"
        n160 = Unbundle By Name(w436) -> ("AWG channel name"=w434:string, "AWG resource name"=w437:string)
        n161 = Unbundle By Name(w426) -> ("Duty cycle index"=w425:i32)
        n162 = Unbundle By Name(w436) -> ("AWG source trigger"=w421:string, "PWM frequency"=w432:dbl, "AWG amplitude"=w431:dbl, "AWG dc offset"=w435:dbl, "AWG load impedence"=w423:dbl, "Duty cycle single pulse/sweep pulse"=w430:bool, "Duty cycle single point"=w429:dbl)
        n163 = Unbundle By Name(w426) -> ("Frequency sweep values"=w428:dbl[], "Duty cycle index"=w427:i32)
        n164 = call <instrlib>:"niFgen Initialize With Channels.vi"("error in (no error)"=w450, "Channel Name"=w434, "Resource Name"=w437) -> ("error out"=w452:errorcluster, "Instrument Handle Out"=w451:refnum<k15>)  [unwired: 7 in]
        n165 = call <instrlib>:"niFgen Configure Output Mode.vi"("error in (no error)"=w452, "Output Mode (default: 0=Standard Function)"=w453, "Instrument Handle"=w451) -> ("error out"=w455:errorcluster, "Instrument Handle Out"=w454:refnum<k15>)  [unwired: 6 in]
        n166 = case shown="True" w430 {
          tunnel: w429 -> [w456 _]
          tunnel: [w456 w457] -> w422
          tunnel: w428 -> [_ w459]
          tunnel: w427 -> [_ w458]
          frame False {
          }
          frame True {
            n167 = Index Array(array=w459, index=w458) -> (element=w457:dbl)
          }
        }
        n168 = call <instrlib>:"niFgen Configure Standard Waveform.vi"("Instrument Handle"=w454, "Channel Name"=w434, "Waveform"=w449, "Frequency"=w432, "Amplitude"=w431, "error in (no error)"=w455, "DC Offset"=w435) -> ("Instrument Handle Out"=w448:refnum<k15>, "error out"=w438:errorcluster)  [unwired: 7 in]
        n169 = property class="niFgen"(reference=w448, error in=w438, "Load Impedance"=w423, "Duty Cycle High"=w422) -> (reference out=w447:refnum<k15>, error out=w446:errorcluster)
        n170 = call-poly <instrlib>:"niFgen Configure Trigger (poly).vi"("error in (no error)"=w446, "Source"=w421, "Instrument Handle"=w447) -> ("error out"=w444:errorcluster, "Instrument Handle Out"=w445:refnum<k15>)  [unwired: 7 in]
        n171 = call <instrlib>:"niFgen Output Enable.vi"("error in (no error)"=w444, "Output Enable (default: True)"=TRUE ("output enable"), "Channel Name"=w434, "Instrument Handle"=w445) -> ("error out"=w442:errorcluster, "Instrument Handle Out"=w441:refnum<k15>)  [unwired: 6 in]
        n172 = Increment(x=w425) -> (x+1=w424:i32)
        n173 = call <instrlib>:"niFgen Initiate Generation.vi"("error in (no error)"=w442, "Instrument Handle"=w441) -> ("error out"=w439:errorcluster, "Instrument Handle Out"=w440:refnum<k15>)  [unwired: 8 in]
        n174 = Bundle By Name(cluster=w426, "Duty cycle index"=w424, "AWG Out"=w440, "Frequency"=w432, "PWM voltage level"=w431) -> (w443:T3)
      }
      frame "InitializeScope" {
        w486 = 2 items=["None"=1, "Auto Trigger"=2] ("Trigger Modifier")
        w480 = u32 0 items=["1 mega ohm"=0, "50 ohms"=2] ("Input Impedance")
        w483 = T11 0 items=["Positive", "Negative"] ("trigger slope")
        # "Initializing scope for measureing inpu voltage for calculating input duty cycle"
        n175 = Unbundle By Name(w470) -> ("Scope vertical coupling"=w466:enum32{"AC", "DC"}, "Scope probe attenuation"=w467:dbl, "Scope input channel name"=w468:string, "Scope resource name"=w469:string)  [unwired: 1 out]
        n176 = Unbundle By Name(w470) -> ("Scope vertical range"=w471:dbl, "Scope sample rate"=w464:dbl, "Duty cycle single pulse/sweep pulse"=w463:bool)
        n177 = Unbundle By Name(w465) -> ("No of samples to fetch scope single"=w462:i32, "No of samples to fetch scope"=w460:i32)
        n178 = call <instrlib>:"niScope Initialize With Options.vi"("resource name"=w469, "error in"=w477) -> ("instrument handle"=w497:refnum<k15>, "error out"=w496:errorcluster)  [unwired: 12 in]
        n179 = call-poly <instrlib>:"niScope Get Channel Name (Poly).vi"("instrument handle"=w497, "index"=w468, "error in"=w496) -> ("instrument handle out"=w485:refnum<k15>, "channel name"=w481:string, "error out"=w484:errorcluster)  [unwired: 10 in]
        n180 = Select(t=w462, s=w463, f=w460) -> (s? t:f=w461:i32)
        n181 = call <instrlib>:"niScope Configure Vertical.vi"("instrument handle"=w485, "probe attenuation"=w467, "vertical coupling"=w466, "channels"=w481, "vertical range"=w471, "vertical offset"=0.0, "error in"=w484) -> ("instrument handle out"=w495:refnum<k15>, "error out"=w494:errorcluster)  [unwired: 7 in]
        n182 = call <instrlib>:"niScope Configure Chan Characteristics.vi"("instrument handle"=w495, "channels"=w481, "input impedance"=w480, "maximum input frequency"=-1.0 ("Maximum Input Frequency"), "error in"=w494) -> ("instrument handle out"=w492:refnum<k15>, "error out"=w493:errorcluster)  [unwired: 9 in]
        n183 = call <instrlib>:"niScope Configure Horizontal Timing.vi"("instrument handle"=w492, "min sample rate"=w464, "reference position"=0.0 ("Reference Position"), "error in"=w493, "min record length"=w461) -> ("instrument handle out"=w489:refnum<k15>, "error out"=w488:errorcluster)  [unwired: 9 in]
        n184 = Unbundle By Name(w465) -> ("Measure trigger terminal measure"=w482:string)
        n185 = property on="Property Node" class="niScope"(reference=w489, error in=w488, "Trigger Modifier"=w486) -> (reference out=w478:refnum<k15>, error out=w487:errorcluster)
        n186 = call-poly <instrlib>:"niScope Configure Trigger (poly).vi"("instrument handle"=w478, "trigger slope"=w483, "trigger source"=w482, "error in"=w487) -> ("instrument handle out"=w475:refnum<k15>, "error out"=w472:errorcluster)  [unwired: 10 in]
        n187 = call <instrlib>:"niScope Initiate Acquisition.vi"("instrument handle"=w475, "error in"=w472) -> ("instrument handle out"=w474:refnum<k15>, "error out"=w473:errorcluster)  [unwired: 12 in]
        n188 = Bundle By Name(cluster=w465, "scope channel name"=w481, "scope instrument handle out"=w474, "Scope sample rate"=w464) -> (w476:T3)
      }
      frame "PerformMeasurementSingleCycle" {
        w501 = dbl[] [] ("Measurement Results.Input duty cycle(%)")
        w505 = T4 1051 items=["Source Complete Event"=1030, "Measure Complete Event"=1031, "Sequence Iteration Complete Event"=1032, "Sequence Engine Done Event"=1033, "Pulse Complete Event"=1051, "Ready For Pulse Trigger Event"=1052] ("event")
        # "1.Fetches the voltages and currents of both the PPS and E-Load as per numbers of samples fetched"
        # "Capturing the results from source, load and scope"
        n189 = Unbundle By Name(w529) -> ("No of samples to fetch smu"=w504:i32, "Load channel name"=w502:string, "Load out"=w503:refnum<k15>)
        n190 = Unbundle By Name(w529) -> ("Source out"=w522:refnum<k15>, "Source channel name"=w521:string, "No of samples to fetch smu"=w520:i32, "scope instrument handle out"=w528:refnum<k15>, "scope channel name"=w527:string, "No of samples to fetch scope"=w526:i32)
        n191 = Unbundle By Name(w500) -> ("Measurement timeout"=w498:dbl)
        n192 = call <instrlib>:"niDCPower Initiate With Channels.vi"("error in (no error)"=w507, "channel name"=w502, "instrument handle"=w503) -> ("error out"=w510:errorcluster, "instrument handle out"=w509:refnum<k15>)  [unwired: 7 in]
        n193 = call <instrlib>:"niDCPower Wait For Event With Channels.vi"("error in (no error)"=w510, "event"=w505, "channel name"=w502, "instrument handle"=w509) -> ("error out"=w506:errorcluster, "instrument handle out"=w508:refnum<k15>)  [unwired: 6 in]
        n194 = call <instrlib>:"niDCPower Fetch Multiple.vi"("instrument handle"=w508, "channel name"=w502, "count (1)"=w504, "timeout (1.0)"=w498, "error in (no error)"=w506) -> ("instrument handle out"=w525:refnum<k15>, "voltage measurements"=w519:dbl[], "current measurements"=w517:dbl[], "error out"=w499:errorcluster)  [unwired: 5 in, 2 out]
        n195 = call <instrlib>:"niDCPower Fetch Multiple.vi"("instrument handle"=w522, "channel name"=w521, "count (1)"=w520, "timeout (1.0)"=w498, "error in (no error)"=w499) -> ("instrument handle out"=w516:refnum<k15>, "voltage measurements"=w515:dbl[], "error out"=w523:errorcluster)  [unwired: 5 in, 3 out]
        n196 = call-poly <instrlib>:"niScope Fetch (poly).vi"("error in"=w523, "numSamples"=w526, "channels"=w527, "instrument handle"=w528) -> ("error out"=w524:errorcluster, "wfm"=w513:waveform(dbl), "instrument handle out"=w514:refnum<k15>)  [unwired: 4 in, 1 out]
        n197 = Absolute Value(x=w517) -> (abs(x)=w518:dbl[])
        n198 = Unbundle By Name(w513) -> ("Y"=w512:dbl[], "dt"=w511:dbl)
        n199 = Bundle By Name(cluster=w529, "Load out"=w525, "Measurement Results.Output voltages(SMU)"=w519, "Measurement Results.Output currents(SMU)"=w518, "Source out"=w516, "Measurement Results.Input voltages(SMU)"=w515, "scope instrument handle out"=w514, "Measurement Results.PWM input voltage(scope amplitude)"=w512, "Measurement Results.Scope dt"=w511, "Measurement Results.Input duty cycle(%)"=w501, "Measurement Results.Output duty cycle(%)"=w501) -> (w530:T3)
      }
      frame "PerformMeasurementSweepCycle" {
        w546 = T4 1030 items=["Source Complete Event"=1030, "Measure Complete Event"=1031, "Sequence Iteration Complete Event"=1032, "Sequence Engine Done Event"=1033, "Pulse Complete Event"=1051, "Ready For Pulse Trigger Event"=1052] ("event")
        # "Capturing the results from source, load and scope and also calculating duty cycle for input voltage from AWG and output current from load"
        n200 = Unbundle By Name(w563) -> ("Measurement Results.Output voltages(SMU)"=w562:dbl[], "Measurement Results.Output currents(SMU)"=w561:dbl[], "Measurement Results.Input voltages(SMU)"=w560:dbl[], "Measurement Results.PWM input voltage(scope amplitude)"=w559:dbl[])
        n201 = Unbundle By Name(w563) -> ("No of samples to fetch smu single"=w550:i32, "Load channel name"=w547:string, "Load out"=w548:refnum<k15>)
        n202 = Unbundle By Name(w563) -> ("Source out"=w579:refnum<k15>, "Source channel name"=w578:string, "No of samples to fetch smu single"=w577:i32, "scope instrument handle out"=w584:refnum<k15>, "scope channel name"=w583:string, "No of samples to fetch scope single"=w582:i32)
        n203 = Unbundle By Name(w545) -> ("Measurement timeout"=w544:dbl)
        n204 = call <instrlib>:"niDCPower Initiate With Channels.vi"("error in (no error)"=w552, "channel name"=w547, "instrument handle"=w548) -> ("error out"=w554:errorcluster, "instrument handle out"=w553:refnum<k15>)  [unwired: 7 in]
        n205 = call <instrlib>:"niDCPower Wait For Event With Channels.vi"("error in (no error)"=w554, "event"=w546, "channel name"=w547, "instrument handle"=w553) -> ("error out"=w551:errorcluster, "instrument handle out"=w549:refnum<k15>)  [unwired: 6 in]
        n206 = call <instrlib>:"niDCPower Fetch Multiple.vi"("instrument handle"=w549, "channel name"=w547, "count (1)"=w550, "timeout (1.0)"=w544, "error in (no error)"=w551) -> ("instrument handle out"=w567:refnum<k15>, "voltage measurements"=w575:dbl[], "current measurements"=w565:dbl[], "error out"=w581:errorcluster)  [unwired: 5 in, 2 out]
        n207 = Absolute Value(x=w565) -> (abs(x)=w534:dbl[])
        n208 = call <instrlib>:"niDCPower Fetch Multiple.vi"("instrument handle"=w579, "channel name"=w578, "count (1)"=w577, "timeout (1.0)"=w544, "error in (no error)"=w581) -> ("instrument handle out"=w571:refnum<k15>, "voltage measurements"=w574:dbl[], "error out"=w580:errorcluster)  [unwired: 5 in, 3 out]
        n209 = call-poly <instrlib>:"niScope Fetch (poly).vi"("error in"=w580, "numSamples"=w582, "channels"=w583, "instrument handle"=w584) -> ("error out"=w538:errorcluster, "wfm"=w576:waveform(dbl), "instrument handle out"=w566:refnum<k15>)  [unwired: 4 in, 1 out]
        n210 = Unbundle By Name(w563) -> ("Current level absolute"=w533:dbl, "Load sample rate"=w532:dbl, "Frequency"=w531:dbl, "Measurement Results.Output duty cycle(%)"=w557:dbl[], "Measurement Results.Input duty cycle(%)"=w558:dbl[], "PWM voltage level"=w541:dbl, "Scope sample rate"=w540:dbl, "Frequency"=w539:dbl)
        n211 = Unbundle By Name(w576) -> ("Y"=w542:dbl[], "dt"=w568:dbl)
        n212 = call "Calculate Duty Cycle.vi"("Voltage/Current Values"=w534, "Pulse voltage/Current level"=w533, "Sample rate"=w532, "Frequency"=w531, "error in"=w538) -> ("Duty Cycle"=w535:dbl, "error out"=w537:errorcluster)  [unwired: 9 in]
        n213 = Build Array (concatenate)(w559, w542) -> (w569:dbl[])
        n214 = Build Array (concatenate)(w562, w575) -> (w573:dbl[])
        n215 = Build Array (concatenate)(w561, w534) -> (w572:dbl[])
        n216 = Build Array (concatenate)(w560, w574) -> (w570:dbl[])
        n217 = call "Calculate Duty Cycle.vi"("Voltage/Current Values"=w542, "Pulse voltage/Current level"=w541, "Sample rate"=w540, "Frequency"=w539, "error in"=w537) -> ("Duty Cycle"=w543:dbl, "error out"=w536:errorcluster)  [unwired: 9 in]
        n218 = Build Array (concatenate)(w557, w535) -> (w556:dbl[])
        n219 = Build Array (concatenate)(w558, w543) -> (w555:dbl[])
        n220 = Bundle By Name(cluster=w563, "Load out"=w567, "Measurement Results.Output voltages(SMU)"=w573, "Measurement Results.Output currents(SMU)"=w572, "Source out"=w571, "Measurement Results.Input voltages(SMU)"=w570, "scope instrument handle out"=w566, "Measurement Results.PWM input voltage(scope amplitude)"=w569, "Measurement Results.Scope dt"=w568, "Measurement Results.Input duty cycle(%)"=w556, "Measurement Results.Output duty cycle(%)"=w555) -> (w564:T3)
      }
      frame "CloseSessionsforSweeps" {
        # "Aborting smu session beacuse same session can be used again closing and aboritng fgen genearting and scope as we cannot use same session againg for next duty cycle"
        n221 = Unbundle By Name(w596) -> ("scope instrument handle out"=w586:refnum<k15>, "AWG Out"=w587:refnum<k15>, "Load out"=w589:refnum<k15>, "Load channel name"=w588:string, "Source out"=w593:refnum<k15>, "Source channel name"=w592:string)
        n222 = call <instrlib>:"niDCPower Abort With Channels.vi"("error in (no error)"=w585, "channel name"=w592, "instrument handle"=w593) -> ("error out"=w600:errorcluster, "instrument handle out"=w595:refnum<k15>)  [unwired: 7 in]
        n223 = call <instrlib>:"niDCPower Abort With Channels.vi"("error in (no error)"=w600, "channel name"=w588, "instrument handle"=w589) -> ("error out"=w601:errorcluster, "instrument handle out"=w594:refnum<k15>)  [unwired: 7 in]
        n224 = call <instrlib>:"niFgen Abort Generation.vi"("error in (no error)"=w601, "Instrument Handle"=w587) -> ("error out"=w599:errorcluster, "Instrument Handle Out"=w597:refnum<k15>)  [unwired: 8 in]
        n225 = call <instrlib>:"niFgen Close.vi"("error in (no error)"=w599, "Instrument Handle"=w597) -> ("error out"=w598:errorcluster)  [unwired: 9 in]
        n226 = call <instrlib>:"niScope Close.vi"("instrument handle"=w586, "error in"=w598) -> ("error out"=w591:errorcluster)  [unwired: 13 in]
        n227 = Bundle By Name(cluster=w596, "Source out"=w595, "Load out"=w594) -> (w590:T3)
      }
      frame "Exit" {
        # "Closing all the session for both single point and sweep duty cycle"
        n228 = Release Queue(queue=w608, error in (no error)=w607) -> (error out=w606:errorcluster)  [unwired: 1 in, 2 out]
        n229 = Unbundle By Name(w603) -> ("Duty cycle single pulse/sweep pulse"=w602:bool)
        n230 = case shown="True" w602 {
          tunnel: w606 -> [w610 w659]
          tunnel: w604 -> [w611 w661]
          tunnel: [w612 w660] -> w605
          frame False {
            n231 = case shown="Error .." w610 {
              selector: w610 -> [w613 w636]
              tunnel: [w624 w637] -> w612
              tunnel: w611 -> [w614 w639]
              frame No Error {
                n232 = Unbundle By Name(w614) -> ("scope instrument handle out"=w625:refnum<k15>, "AWG Out"=w626:refnum<k15>, "Source out"=w619:refnum<k15>, "Source channel name"=w618:string, "Load out"=w623:refnum<k15>, "Load channel name"=w622:string)
                n233 = call <instrlib>:"niDCPower Abort With Channels.vi"("error in (no error)"=w613, "channel name"=w622, "instrument handle"=w623) -> ("error out"=w621:errorcluster, "instrument handle out"=w620:refnum<k15>)  [unwired: 7 in]
                n234 = call <instrlib>:"niDCPower Reset.vi"("error in (no error)"=w621, "instrument handle"=w620) -> ("error out"=w631:errorcluster, "instrument handle out"=w634:refnum<k15>)  [unwired: 2 in, 6 out]
                n235 = call <instrlib>:"niDCPower Close.vi"("error in (no error)"=w631, "instrument handle"=w634) -> ("error out"=w617:errorcluster)  [unwired: 9 out]
                n236 = call <instrlib>:"niDCPower Abort With Channels.vi"("error in (no error)"=w617, "channel name"=w618, "instrument handle"=w619) -> ("error out"=w616:errorcluster, "instrument handle out"=w615:refnum<k15>)  [unwired: 7 in]
                n237 = call <instrlib>:"niDCPower Reset.vi"("error in (no error)"=w616, "instrument handle"=w615) -> ("error out"=w633:errorcluster, "instrument handle out"=w632:refnum<k15>)  [unwired: 2 in, 6 out]
                n238 = call <instrlib>:"niDCPower Close.vi"("error in (no error)"=w633, "instrument handle"=w632) -> ("error out"=w627:errorcluster)  [unwired: 9 out]
                n239 = call <instrlib>:"niFgen Abort Generation.vi"("error in (no error)"=w627, "Instrument Handle"=w626) -> ("error out"=w630:errorcluster, "Instrument Handle Out"=w628:refnum<k15>)  [unwired: 8 in]
                n240 = call <instrlib>:"niFgen Close.vi"("error in (no error)"=w630, "Instrument Handle"=w628) -> ("error out"=w629:errorcluster)  [unwired: 9 in]
                n241 = call <instrlib>:"niScope Close.vi"("instrument handle"=w625, "error in"=w629) -> ("error out"=w624:errorcluster)  [unwired: 13 in]
              }
              frame Error {
                n242 = Unbundle By Name(w639) -> ("scope instrument handle out"=w638:refnum<k15>, "AWG Out"=w650:refnum<k15>, "Source out"=w645:refnum<k15>, "Source channel name"=w644:string, "Load out"=w649:refnum<k15>, "Load channel name"=w648:string)
                n243 = call <vilib>:"Clear Errors.vi"("error in (no error)"=w636) -> ("error out"=w640:errorcluster)  [unwired: 5 in, 1 out]
                n244 = call <instrlib>:"niDCPower Abort With Channels.vi"("error in (no error)"=w640, "channel name"=w648, "instrument handle"=w649) -> ("error out"=w647:errorcluster, "instrument handle out"=w646:refnum<k15>)  [unwired: 7 in]
                n245 = call <instrlib>:"niDCPower Reset.vi"("error in (no error)"=w647, "instrument handle"=w646) -> ("error out"=w655:errorcluster, "instrument handle out"=w658:refnum<k15>)  [unwired: 2 in, 6 out]
                n246 = call <instrlib>:"niDCPower Close.vi"("error in (no error)"=w655, "instrument handle"=w658) -> ("error out"=w643:errorcluster)  [unwired: 9 out]
                n247 = call <instrlib>:"niDCPower Abort With Channels.vi"("error in (no error)"=w643, "channel name"=w644, "instrument handle"=w645) -> ("error out"=w642:errorcluster, "instrument handle out"=w641:refnum<k15>)  [unwired: 7 in]
                n248 = call <instrlib>:"niDCPower Reset.vi"("error in (no error)"=w642, "instrument handle"=w641) -> ("error out"=w657:errorcluster, "instrument handle out"=w656:refnum<k15>)  [unwired: 2 in, 6 out]
                n249 = call <instrlib>:"niDCPower Close.vi"("error in (no error)"=w657, "instrument handle"=w656) -> ("error out"=w651:errorcluster)  [unwired: 9 out]
                n250 = call <instrlib>:"niFgen Abort Generation.vi"("error in (no error)"=w651, "Instrument Handle"=w650) -> ("error out"=w654:errorcluster, "Instrument Handle Out"=w652:refnum<k15>)  [unwired: 8 in]
                n251 = call <instrlib>:"niFgen Close.vi"("error in (no error)"=w654, "Instrument Handle"=w652) -> ("error out"=w653:errorcluster)  [unwired: 9 in]
                n252 = call <instrlib>:"niScope Close.vi"("instrument handle"=w638, "error in"=w653) -> ("error out"=w635:errorcluster)  [unwired: 13 in]
                n253 = Merge Errors(w635, w636) -> (w637:errorcluster)
              }
            }
          }
          frame True {
            n254 = case shown="Error .." w659 {
              selector: w659 -> [w662 w673]
              tunnel: w661 -> [w671 w676]
              tunnel: [w670 w672] -> w660
              frame No Error {
                n255 = Unbundle By Name(w671) -> ("Source out"=w663:refnum<k15>, "Load out"=w669:refnum<k15>)
                n256 = call <instrlib>:"niDCPower Reset.vi"("error in (no error)"=w662, "instrument handle"=w669) -> ("error out"=w664:errorcluster, "instrument handle out"=w668:refnum<k15>)  [unwired: 2 in, 6 out]
                n257 = call <instrlib>:"niDCPower Close.vi"("error in (no error)"=w664, "instrument handle"=w668) -> ("error out"=w667:errorcluster)  [unwired: 9 out]
                n258 = call <instrlib>:"niDCPower Reset.vi"("error in (no error)"=w667, "instrument handle"=w663) -> ("error out"=w666:errorcluster, "instrument handle out"=w665:refnum<k15>)  [unwired: 2 in, 6 out]
                n259 = call <instrlib>:"niDCPower Close.vi"("error in (no error)"=w666, "instrument handle"=w665) -> ("error out"=w670:errorcluster)  [unwired: 9 out]
              }
              frame Error {
                n260 = Unbundle By Name(w676) -> ("scope instrument handle out"=w686:refnum<k15>, "AWG Out"=w687:refnum<k15>, "Source out"=w681:refnum<k15>, "Source channel name"=w680:string, "Load out"=w685:refnum<k15>, "Load channel name"=w684:string)
                n261 = call <vilib>:"Clear Errors.vi"("error in (no error)"=w673) -> ("error out"=w675:errorcluster)  [unwired: 5 in, 1 out]
                n262 = call <instrlib>:"niDCPower Abort With Channels.vi"("error in (no error)"=w675, "channel name"=w684, "instrument handle"=w685) -> ("error out"=w683:errorcluster, "instrument handle out"=w682:refnum<k15>)  [unwired: 7 in]
                n263 = call <instrlib>:"niDCPower Reset.vi"("error in (no error)"=w683, "instrument handle"=w682) -> ("error out"=w692:errorcluster, "instrument handle out"=w695:refnum<k15>)  [unwired: 2 in, 6 out]
                n264 = call <instrlib>:"niDCPower Close.vi"("error in (no error)"=w692, "instrument handle"=w695) -> ("error out"=w679:errorcluster)  [unwired: 9 out]
                n265 = call <instrlib>:"niDCPower Abort With Channels.vi"("error in (no error)"=w679, "channel name"=w680, "instrument handle"=w681) -> ("error out"=w678:errorcluster, "instrument handle out"=w677:refnum<k15>)  [unwired: 7 in]
                n266 = call <instrlib>:"niDCPower Reset.vi"("error in (no error)"=w678, "instrument handle"=w677) -> ("error out"=w694:errorcluster, "instrument handle out"=w693:refnum<k15>)  [unwired: 2 in, 6 out]
                n267 = call <instrlib>:"niDCPower Close.vi"("error in (no error)"=w694, "instrument handle"=w693) -> ("error out"=w688:errorcluster)  [unwired: 9 out]
                n268 = call <instrlib>:"niFgen Abort Generation.vi"("error in (no error)"=w688, "Instrument Handle"=w687) -> ("error out"=w691:errorcluster, "Instrument Handle Out"=w689:refnum<k15>)  [unwired: 8 in]
                n269 = call <instrlib>:"niFgen Close.vi"("error in (no error)"=w691, "Instrument Handle"=w689) -> ("error out"=w690:errorcluster)  [unwired: 9 in]
                n270 = call <instrlib>:"niScope Close.vi"("instrument handle"=w686, "error in"=w690) -> ("error out"=w674:errorcluster)  [unwired: 13 in]
                n271 = Merge Errors(w674, w673) -> (w672:errorcluster)
              }
            }
          }
        }
      }
    }
  }
  "error out" <- w25
  n272 = Unbundle By Name(w17) -> ("Measurement Results"=→"measurement results":T1)
  "measure call context out" <- "measure call context in"
